vi "运维调试_总磷总氮.vi"() -> ()   [LabVIEW 2016, in "斯坦道总磷总氮.lvlib"]
uses:
  <vilib>/Utility/miscctls.llb/LVPointTypeDef.ctl
  <vilib>/Utility/config.llb/NI_LVConfig.lvlib
  <vilib>/ptbypt/NI_PtbyPt.lvlib
panel:
  in  "定时设置":cluster{"启动":bool, "控制命令":T1, "测量参数":T2}(xcontrol)
  in  "总磷参数设置":bool
  in  "总氮参数设置":bool
  in  "模块启用":bool
  in  "串口设置":bool
  in  "备用系数一键写入":bool
  in  "公式一键写入":bool
  in  "流程路径":path=path "C:/Users/std/Documents/斯坦道流程文件/流程.xml"
  in  "曲线模型":cluster{"X^2":dbl, "X":dbl, "B":dbl, "r^2":dbl}(xcontrol)
  out "字符串 2":string
  in  "质控参数设置":bool
  in  "总氮自动测试量程配置":T3
  in  "总磷自动测试量程配置":T3
  out "温度2":sgl
  out "温度1":sgl
  out "ADC":sgl
  out "固件版本号":string
  in  "数组":string[](array[string])
  in  "备用系数写入":bool
  in  "备用系数读取":bool
  in  "备用系数":T4
  in  "量程切换阈值写入":bool
  in  "量程切换阈值读取":bool
  in  "量程切换阈值":cluster{"阈值":dbl, "标液浓度":dbl}
  in  "参数下拉列表":enum16{"总磷", "总氮"}(ring)
  in  "量程下拉列表":enum16{"低量程", "高量程"}(ring)
  in  "测量模式下拉列表":enum16{"水样测量", "零点核查", "跨度核查", "标样核查", "加标回收"}(ring)
  in  "公式":cluster{"X^2":dbl, "X":dbl, "b":dbl}
  in  "写公式":bool
  in  "读公式":bool
  in  "返回":bool
  in  "设置":bool
  out "序列号":string="序列号"
  out "总氮测量数据":T5(xcontrol)
  out "总磷测量数据":T5(xcontrol)
  out "集成报警信息":string
  out "总磷总氮运行状态":T6(xcontrol)
  in  "停止":bool
  in  "手动启动":bool
  in  "单步测试":bool
  in  "总磷氨氮调试":u16[](xcontrol)
  out "F3":sgl format="%#.6f"
  out "F2":sgl format="%#.6f"
  out "F1":sgl format="%#.6f"
  out "F0":sgl format="%#.6f"
  out "多列列表框":i32(listbox)
  # "参数设置"
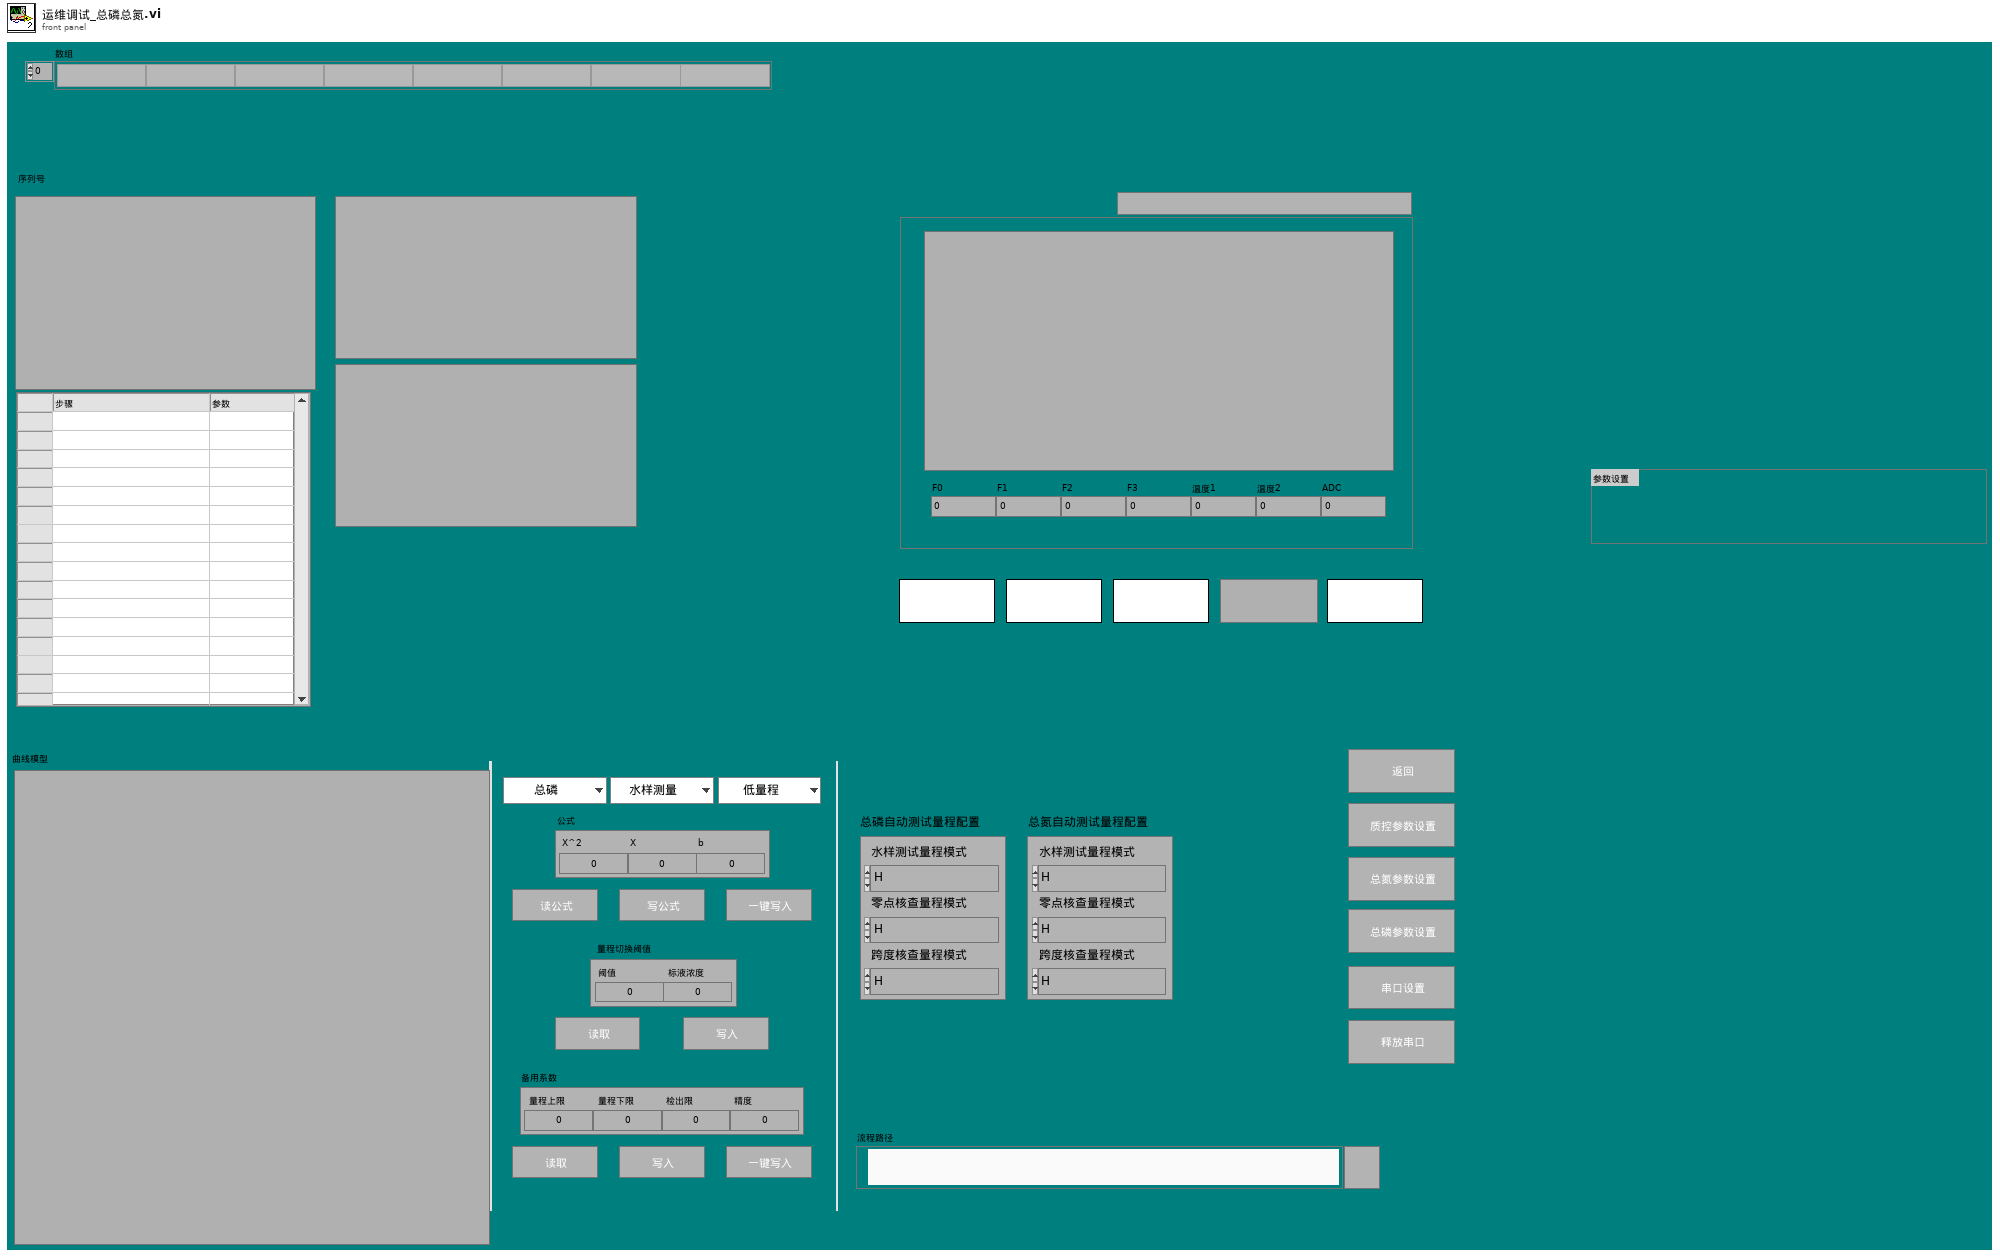
[diagram p1: front panel]
types:
  T1 = typedef "定时设置.xctl/国标控制命令.ctl" = enum16{"启动测量", "标样核查", "零点核查", "跨度核查", "空白测试", "平行样测试", "加标回收", "空白校准", "标样校准", "初始化（清洗）", "停止测试", "仪器重启", "校时", "模式设置", "测量间隔设置"}
  T2 = typedef "定时设置.xctl/测量参数.ctl" = u16
  T3 = cluster{"水样测试量程模式":enum16{"H", "L", "AUTO"}, "空白核查量程模式":enum16{"H", "L", "AUTO"}, "跨度核查量程模式":enum16{"H", "L", "AUTO"}}
  T4 = cluster{"量程上限":dbl, "量程下限":dbl, "检出限":dbl, "精度":dbl}
  T5 = cluster{"flowid":u16, "测量精度":u16, "测量数据区":cluster{"因子编码":u32, "单位":u16, "标样参考值":sgl, "水样数据时间":timestamp, "水样实测值":sgl, "水样数据标识":string, "标样数据时间":timestamp, "标样实测值":sgl, "标样数据标识":string, "空白数据时间":timestamp, "空白实测值":sgl, "空白数据标识":string, "零点核查数据时间":timestamp, "零点核查实测值":sgl, "零点核查数据标识":string, "跨度核查数据时间":timestamp, "跨度核查实测值":sgl, "跨度核查数据标识":string, "加标回收数据时间":timestamp, "加标回收实测值":sgl, "加标回收数据标识":string, "平行样数据时间":timestamp, "平行样实测值":sgl, "平行样数据标识":string, "F0":sgl, "F1":sgl, "F2":sgl, "F3":sgl, "F4":sgl, "F5":sgl, "F6":sgl, "F7":sgl, "温度":sgl, "湿度":sgl, "X值":sgl}}
  T6 = cluster{"系统时间":timestamp, "工作状态":enum16{"空闲", "水样测试", "标样核查", "零点核查", "跨度核查", "空白测试", "平行样测试", "加标回收", "空白校准", "标样校准", "初始化（清洗）"}, "测量模式":enum16{"待机", "连续模式", "周期模式", "定点模式", "受控模式", "手动模式"}, "告警代码":u16, "故障代码":u16, "日志代码":u16, "软件版本":u16, "F0":sgl, "F1":sgl, "F2":sgl, "F3":sgl, "T":sgl, "H":sgl, "id":u16, "flowid":u16, "量程":u16, "总磷控温温度1":sgl, "营养盐控温温度2":sgl, "ADC":sgl}
  T7 = cluster{"时间源选择":enum16{"系统时间源", "仪器时间源"}, "外部时间源":timestamp}
  T8 = enum16{"空闲", "水样测试", "标样核查", "零点核查", "跨度核查", "空白测试", "平行样测试", "加标回收", "空白校准", "标样校准", "初始化（清洗）"}
  T9 = enum32{"Bad", "Idle", "Run top level", "Running"}
  T10 = typedef "定时设置.xctl/周期模式设置.ctl" = enum16{"不启用", "定点模式", "间隔模式"}
  T11 = typedef "定时设置.xctl/定点周期设置.ctl" = cluster{"启动命令":T12, "启动命令 2":T12, "启动命令 3":T12, "启动命令 4":T12, "启动命令 5":T12, "启动命令 6":T12, "启动命令 7":T12, "启动命令 8":T12, "启动命令 9":T12, "启动命令 10":T12, "启动命令 11":T12, "启动命令 12":T12, "启动命令 13":T12, "启动命令 14":T12, "启动命令 15":T12, "启动命令 16":T12, "启动命令 17":T12, "启动命令 18":T12, "启动命令 19":T12, "启动命令 20":T12, "启动命令 21":T12, "启动命令 22":T12, "启动命令 23":T12, "启动命令 24":T12}
  T12 = typedef "定时设置.xctl/启动命令选择.ctl" = u16
  T13 = typedef "定时设置.xctl/间隔启动设置.ctl" = cluster{"启动命令":T12, "启动间隔":dbl, "启动次数":i32}
  T14 = cluster{"周期模式":T10, "定点周期":T11, "间隔启动":T13, "测量参数":T2}
  T15 = typedef "NI_LVConfig.lvlib/Config Data RefNum.ctl" = refnum<k1>
  T16 = typedef "LVPointTypeDef.ctl" = cluster{"Horizontal":i16, "Vertical":i16}
  T17 = cluster{"因子编码":u32, "单位":u16, "标样参考值":sgl, "水样数据时间":timestamp, "水样实测值":sgl, "水样数据标识":string, "标样数据时间":timestamp, "标样实测值":sgl, "标样数据标识":string, "空白数据时间":timestamp, "空白实测值":sgl, "空白数据标识":string, "零点核查数据时间":timestamp, "零点核查实测值":sgl, "零点核查数据标识":string, "跨度核查数据时间":timestamp, "跨度核查实测值":sgl, "跨度核查数据标识":string, "加标回收数据时间":timestamp, "加标回收实测值":sgl, "加标回收数据标识":string, "平行样数据时间":timestamp, "平行样实测值":sgl, "平行样数据标识":string, "F0":sgl, "F1":sgl, "F2":sgl, "F3":sgl, "F4":sgl, "F5":sgl, "F6":sgl, "F7":sgl, "温度":sgl, "湿度":sgl, "X值":sgl}
  T18 = cluster{"参数下拉列表":enum16{"总磷", "总氮"}, "测量模式下拉列表":enum16{"水样测量", "零点核查", "跨度核查", "标样核查", "加标回收"}, "量程下拉列表":enum16{"低量程", "高量程"}}
  T19 = cluster{"启动模式":enum16{"跨度核查", "水样测量", "空白核查", "标样核查", "加标回收"}, "启动参数":u16, "量程":enum16{"低量程", "高量程"}}
  T20 = cluster{"时间标识":timestamp, "设备":string, "日志信息":string, "流程参数":string}
  T21 = cluster{"时间标识":timestamp, "设备":string, "日志信息":string}
  T22 = typedef "LVRowAndColumnUnsignedTypeDef.ctl" = cluster{"Row":u32, "Column":u32}
  T23 = cluster{"站号":u16, "量程切换":enum32{"H", "L", "AUTO"}, "控制命令":enum16{"启动测量", "标样核查", "零点核查", "跨度核查", "空白测试", "平行样测试", "加标回收", "空白校准", "标样校准", "初始化（清洗）", "停止测试", "仪器重启", "校时", "模式设置", "测量间隔设置"}, "模式设置":enum16{"待机", "连续模式", "周期模式", "定点模式", "受控模式", "手动模式"}, "测量间隔":u16}
  T24 = cluster{"总磷跨度值":dbl, "总磷零点标准液浓度":dbl, "总磷跨度标准液浓度":dbl, "总磷标准液标准浓度":dbl, "总氮跨度值":dbl, "总氮零点标准液浓度":dbl, "总氮跨度标准液浓度":dbl, "总氮标准液标准浓度":dbl}
  T25 = cluster{"确定":bool, "总磷跨度值":dbl, "总磷零点标准液浓度":dbl, "总磷跨度标准液浓度":dbl, "总磷标准液标准浓度":dbl, "总氮跨度值":dbl, "总氮零点标准液浓度":dbl, "总氮跨度标准液浓度":dbl, "总氮标准液标准浓度":dbl}
  T26 = cluster{"测量量程":dbl, "测量精度":dbl, "测量间隔":dbl, "消解温度":dbl, "消解时长":dbl, "空白校准时间":timestamp, "曲线截距":dbl, "曲线斜率":dbl, "测量检出限":dbl, "测量信号值":dbl, "线性相关系数":dbl, "二次多项式系数":dbl, "标样校准时间":timestamp, "稀释倍数":dbl, "三项式系数":dbl, "空白标定系数":dbl, "量程系数":dbl, "F0/ORPA":dbl, "F1/ORPB":dbl, "F2/ORPK":dbl, "F3":dbl, "F4":dbl, "F5":dbl, "F6":dbl, "F7":dbl, "X0/滴定数":dbl, "量程":dbl}
  T27 = cluster{"确定":bool, "测量量程":dbl, "测量精度":dbl, "测量间隔":dbl, "消解温度":dbl, "消解时长":dbl, "空白校准时间":timestamp, "曲线截距":dbl, "曲线斜率":dbl, "测量检出限":dbl, "测量信号值":dbl, "线性相关系数":dbl, "二次多项式系数":dbl, "标样校准时间":timestamp, "稀释倍数":dbl, "三项式系数":dbl, "空白标定系数":dbl, "量程系数":dbl, "F0/ORPA":dbl, "F1/ORPB":dbl, "F2/ORPK":dbl, "F3":dbl, "F4":dbl, "F5":dbl, "F6":dbl, "F7":dbl, "X0/滴定数":dbl, "量程":dbl}
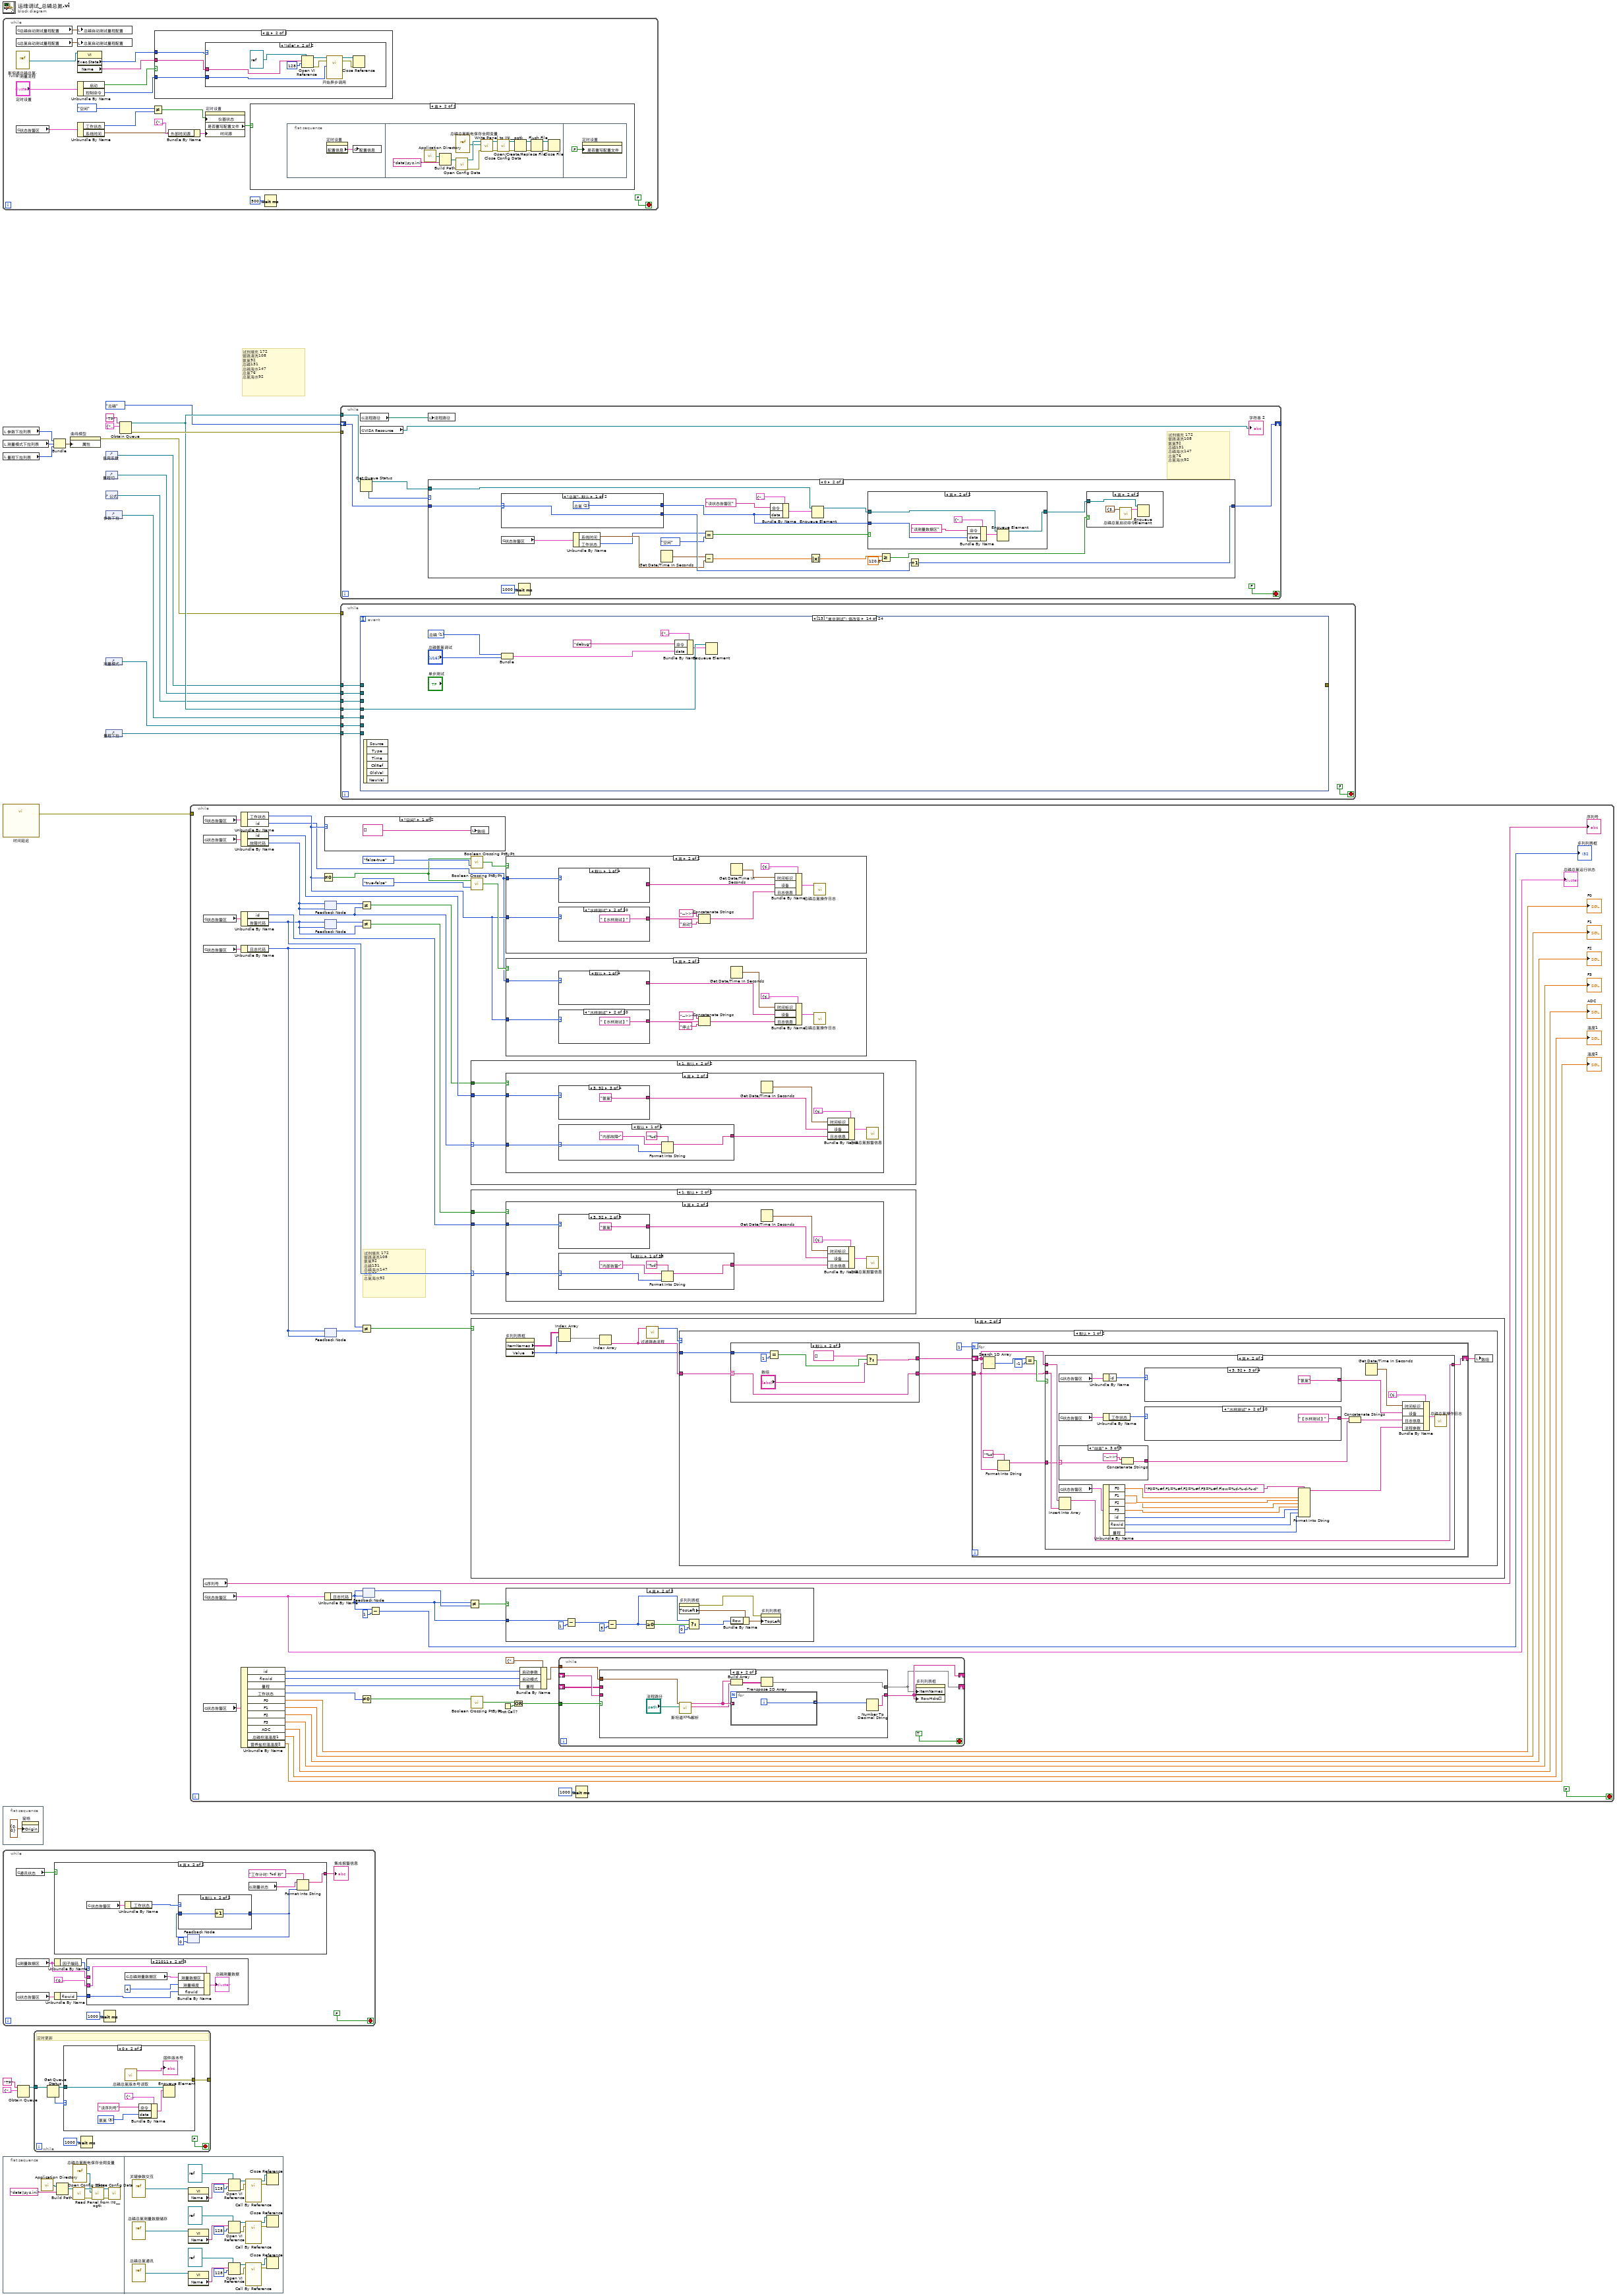
[diagram p0: block diagram]
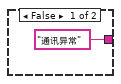
[diagram p3: hidden frame]
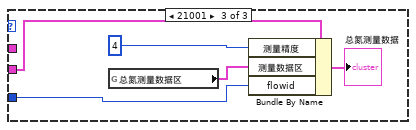
[diagram p6: hidden frame]
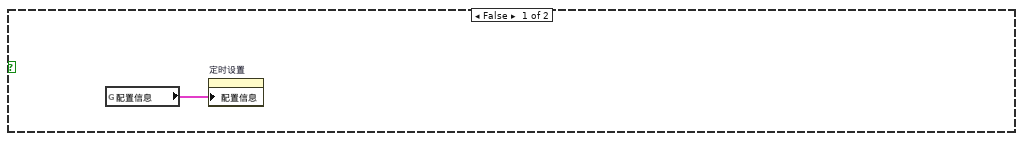
[diagram p7: hidden frame]
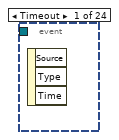
[diagram p10: hidden frame]
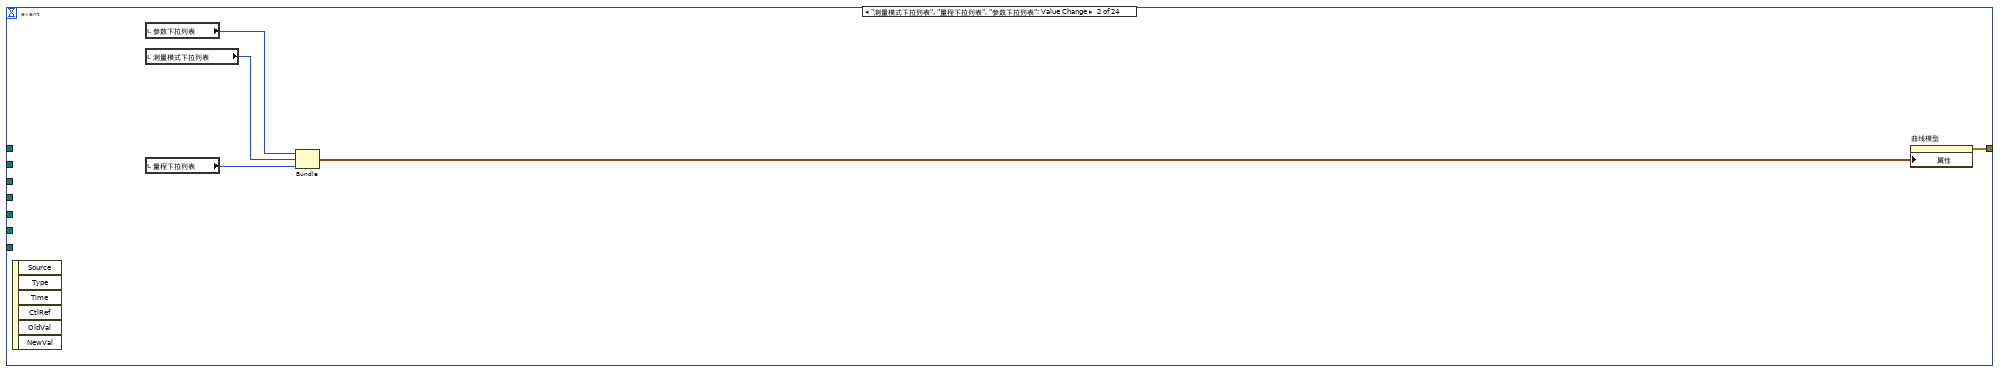
[diagram p11: hidden frame]
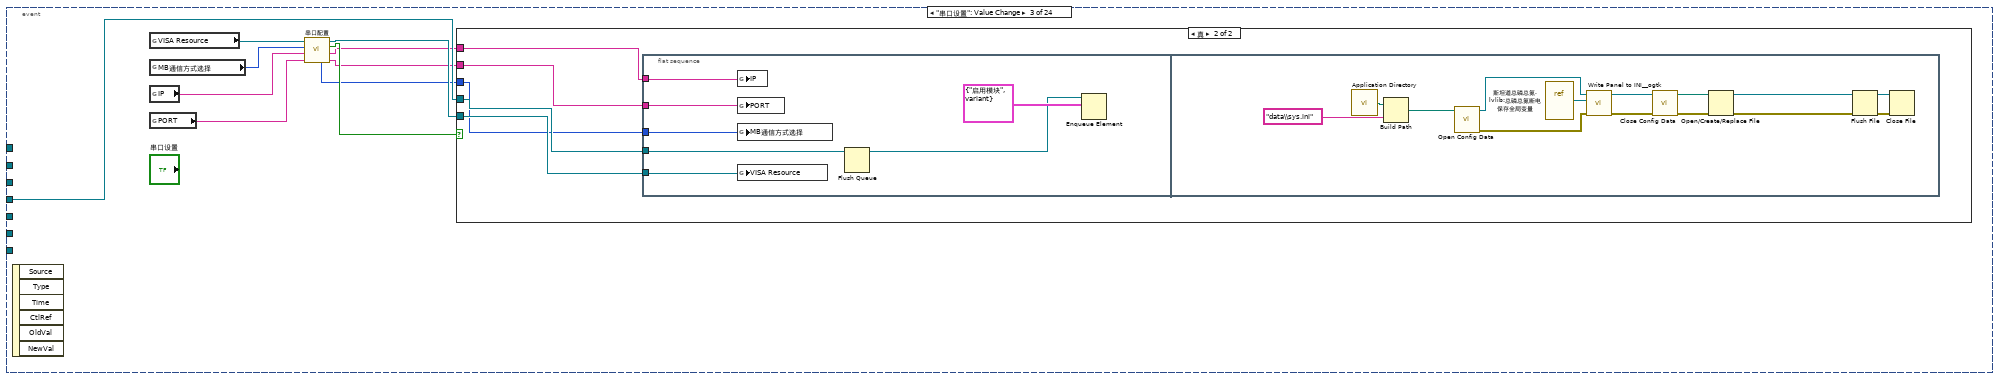
[diagram p12: hidden frame]
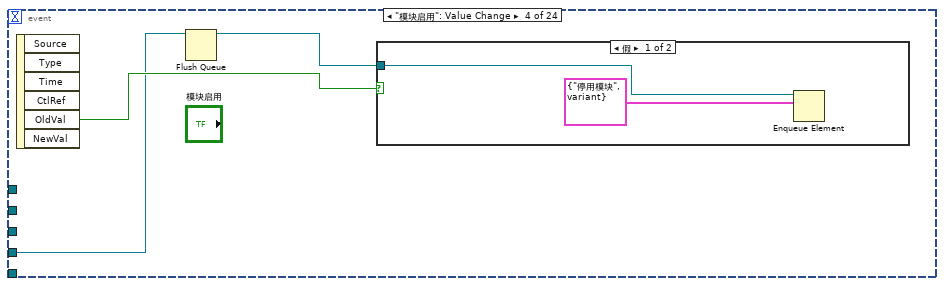
[diagram p14: hidden frame]
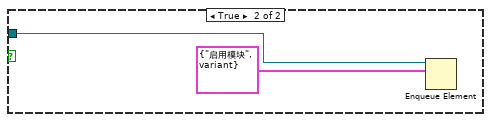
[diagram p15: hidden frame]
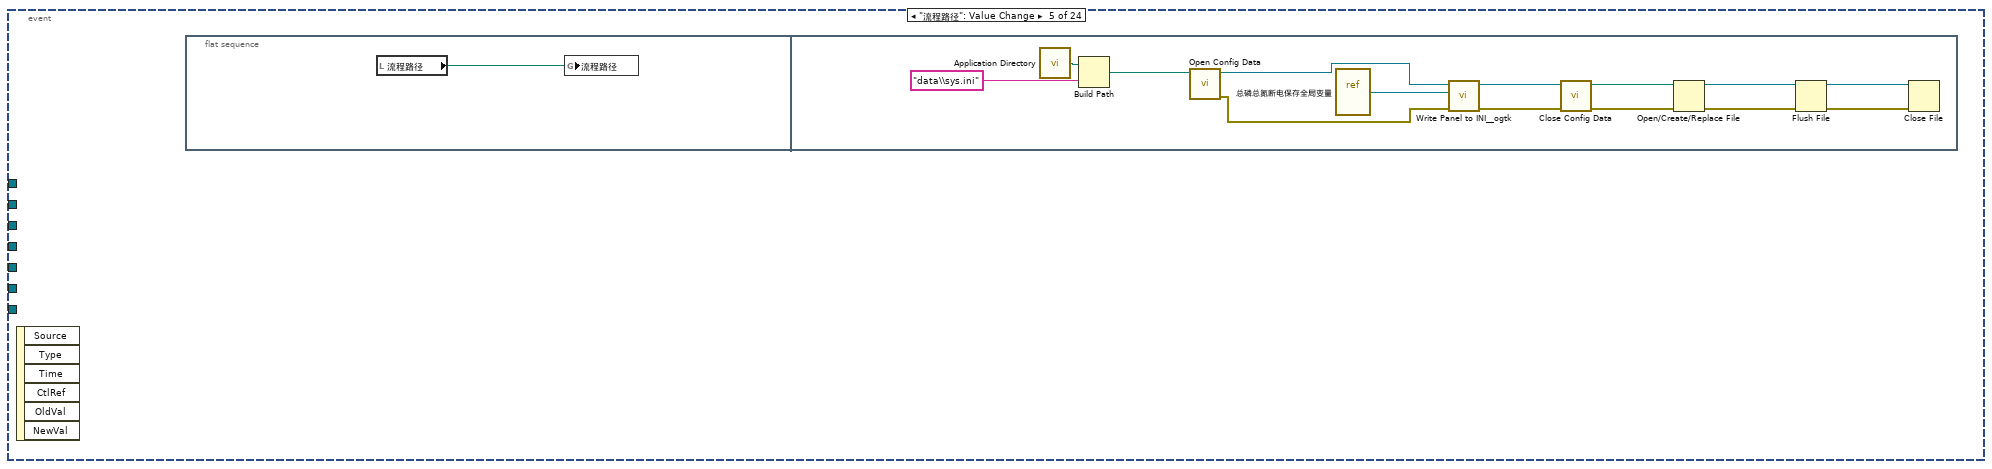
[diagram p16: hidden frame]
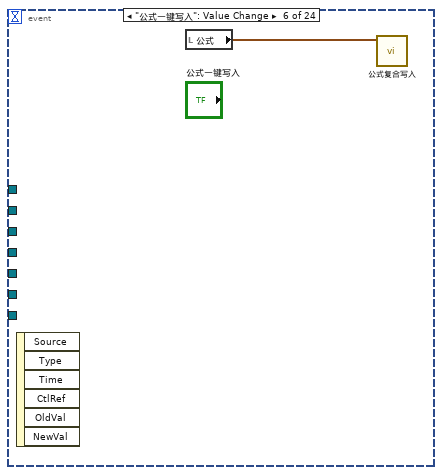
[diagram p17: hidden frame]
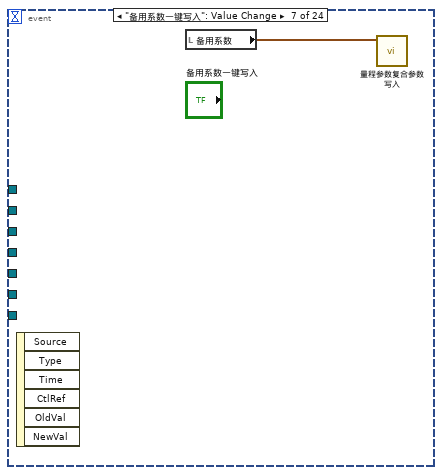
[diagram p18: hidden frame]
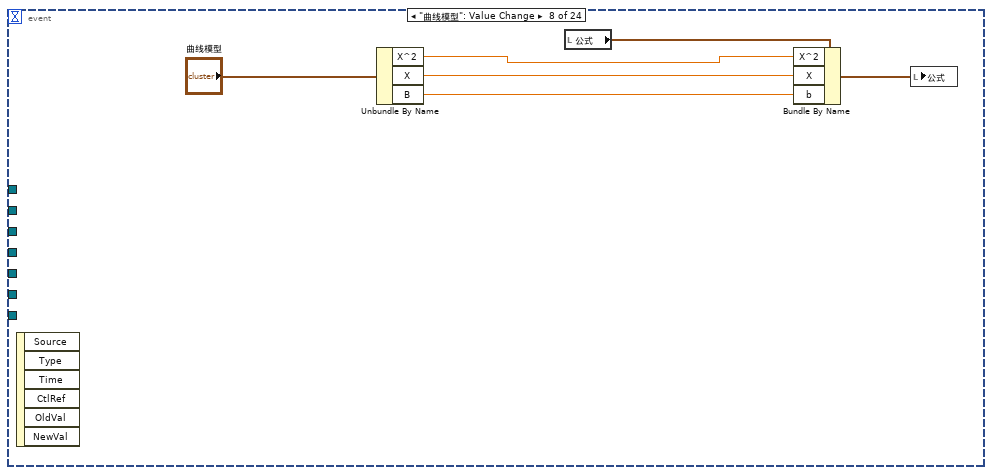
[diagram p19: hidden frame]
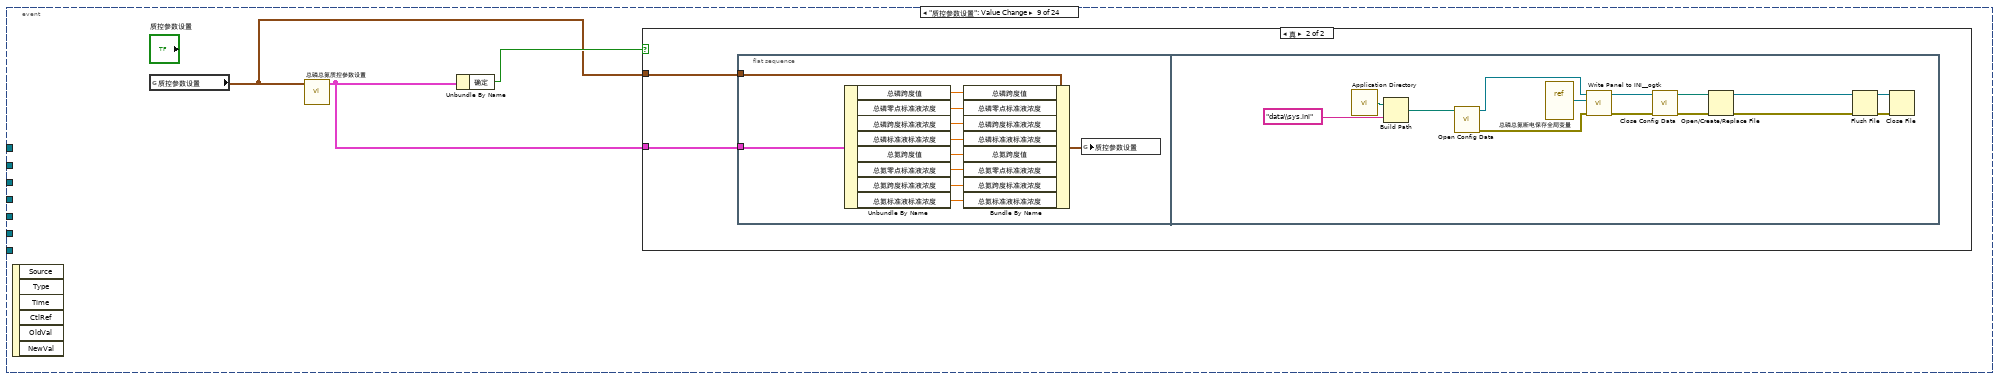
[diagram p20: hidden frame]
diagram:
  # "试剂填充 172 \n管路清洗108\n氨氮92\n总磷131\n总磷海水147\n总氮76\n总氮海水92"
  n1 = while {
    stop <- FALSE stop-if-true
    n2 = global read "总磷总氮断电保存全局变量.vi" "总磷自动测试量程配置"() -> (w35:T3)
    n3 = global read "总磷总氮断电保存全局变量.vi" "总氮自动测试量程配置"() -> (w36:T3)
    n4 = vi-ref "斯坦道总磷总氮.lvlib:测量流程.vi"() -> (w34:refnum<vi>)
    n5 = global read "VAR总磷总氮全局变量.vi" "状态告警区"() -> (w28:T6)
    n6 = local write "总磷自动测试量程配置"(w35) -> ()
    n7 = local write "总氮自动测试量程配置"(w36) -> ()
    n8 = property class="VI"(reference=w34) -> ("Exec.State"=w32:T9, "Name"=w33:string)  [unwired: 1 in, 2 out]
    n9 = Unbundle By Name("定时设置") -> ("启动"=w30:bool, "控制命令"=w29:T1)
    n10 = Unbundle By Name(w28) -> ("工作状态"=w27:T8, "系统时间"=w22:timestamp)
    n11 = Not Equal?(x=T8."空闲", y=w27) -> (x != y?=w25:bool)
    n12 = case shown="真" w30 {
      tunnel: w33 -> [_ w58]
      tunnel: w29 -> [_ w57]
      tunnel: w32 -> [_ w56]
      frame False {
      }
      frame True {
        n13 = case shown="\"Idle\"" w56 {
          tunnel: w58 -> [_ w62]
          tunnel: w57 -> [_ w59]
          frame "Bad", Default {
          }
          frame "Idle" {
            n14 = Open VI Reference(type specifier VI Refnum (for type only)=refnum<vi> refnum, vi path=w62, options=128 ("选项")) -> (vi reference=w63:refnum<vi>, error out=w64:errorcluster)  [unwired: 3 in]
            n15 = call-by-ref "开始异步调用"(reference=w63, error in=w64, "控制命令"=w59) -> (reference out=w65:refnum<vi>, error out=w66:errorcluster)  [unwired: 11 in]
            n16 = Close Reference(reference=w65, error in (no error)=w66) -> ()  [unwired: 1 out]
          }
        }
      }
    }
    n17 = Bundle By Name(cluster=T7 {"时间源选择"=enum."仪器时间源", "外部时间源"=timestamp(0 s since 1904-01-01)} ("时间源"), "外部时间源"=w22) -> (w21:T7)
    n18 = property on="定时设置" class="定时设置 (严格)"("仪器状态"=w25, "时间源"=w21) -> ("是否重写配置文件"=w24:bool)  [unwired: 2 in, 2 out]
    n19 = case shown="真" w24 {
      frame False {
        n20 = global read "总磷总氮断电保存全局变量.vi" "配置信息"() -> (w39:T14)
        n21 = property on="定时设置" class="定时设置 (严格)"("配置信息"=w39) -> ()  [unwired: 2 in, 2 out]
      }
      frame True {
        n22 = flat-sequence {
          frame #0 {
            n23 = property on="定时设置" class="定时设置 (严格)"() -> ("配置信息"=w40:T14)  [unwired: 2 in, 2 out]
            n24 = global write "总磷总氮断电保存全局变量.vi" "配置信息"(w40) -> ()
          }
          frame #1 {
            n25 = call <vilib>:"Application Directory.vi"() -> ("Application Directory"=w54:path)
            n26 = Build Path(base path=w54, name or relative path="data\\sys.ini" ("名称或相对路径")) -> (appended path=w52:path)
            n27 = vi-ref "总磷总氮断电保存全局变量.vi"() -> (w50:refnum<vi>)
            n28 = call <vilib>:"Open Config Data.vi"("configuration file path"=w52) -> ("error out"=w48:errorcluster, "refnum"=w51:T15)  [unwired: 8 in, 1 out]
            n29 = call <userlib>:"Write Panel to INI__ogtk.vi"("error in (no error)"=w48, "VI ref"=w50, "refnum"=w51) -> ("error out"=w47:errorcluster, "refnum out"=w49:T15)  [unwired: 7 in]
            n30 = call <vilib>:"Close Config Data.vi"("error in (no error)"=w47, "refnum"=w49) -> ("error out"=w42:errorcluster, "file path"=w41:path)  [unwired: 8 in]
            n31 = Open/Create/Replace File(file path (use dialog)=w41, error in=w42) -> (refnum out=w45:refnum<file>, error out=w46:errorcluster)  [unwired: 4 in, 1 out]
            n32 = Flush File(refnum=w45, error in=w46) -> (refnum out=w44:refnum<file>, error out=w43:errorcluster)
            n33 = Close File(refnum=w44, error in=w43) -> ()  [unwired: 2 out]
          }
          frame #2 {
            n34 = property on="定时设置" class="定时设置 (严格)"("是否重写配置文件"=FALSE) -> ()  [unwired: 2 in, 2 out]
          }
        }
      }
    }
    n35 = Wait (ms)(milliseconds to wait=u32 500 ("等待时间（毫秒）")) -> ()  [unwired: 1 out]
  }
  n36 = local read "参数下拉列表"() -> (w2:enum16{"总磷", "总氮"})
  n37 = local read "测量模式下拉列表"() -> (w3:enum16{"水样测量", "零点核查", "跨度核查", "标样核查", "加标回收"})
  n38 = local read "量程下拉列表"() -> (w1:enum16{"低量程", "高量程"})
  n39 = call "时间延迟"() -> ("error out"=w9:errorcluster)  [unwired: 11 in]
  n40 = flat-sequence {
    frame #0 {
      n41 = property on="窗格" class="Pane"("Origin"=T16 {"Horizontal"=0, "Vertical"=0} ("原点")) -> ()  [unwired: 2 in, 2 out]
    }
  }
  n42 = while {
    stop <- FALSE stop-if-true
    n43 = global read "VAR总磷总氮全局变量.vi" "通讯状态"() -> (w72:bool)
    n44 = global read "VAR总磷总氮全局变量.vi" "测量数据区"() -> (w74:T17)
    n45 = global read "VAR总磷总氮全局变量.vi" "状态告警区"() -> (w70:T6)
    n46 = case shown="真" w72 {
      tunnel: ["通讯异常" ("集成报警信息") w79] -> w71
      frame False {
      }
      frame True {
        n47 = global read "VAR总磷总氮全局变量.vi" "状态告警区"() -> (w85:T6)
        n48 = Unbundle By Name(w85) -> ("工作状态"=w84:T8)
        n49 = feedback #1(0) -> (w82:i32)
        n50 = case shown="默认" w84 {
          tunnel: w82 -> [_ w87]
          tunnel: [_ w86] -> w80
          frame "空闲" {
          }
          frame Default {
            n51 = Increment(x=w87) -> (x+1=w86:i32)
          }
        }
        n52 = feedback-in #1(w80) -> ()
        n53 = global read "VAR总磷总氮全局变量.vi" "测量状态"() -> (w78:string)
        n54 = Format Into String(format string="工作计时: %d 秒" ("格式字符串"), initial string=w78, w80) -> (resulting string=w79:string)  [unwired: 1 in, 1 out]
      }
    }
    "集成报警信息" <- w71
    n55 = Unbundle By Name(w74) -> ("因子编码"=w73:u32)
    n56 = Unbundle By Name(w70) -> ("flowid"=w69:u16)
    n57 = case shown="21011" w73 {
      tunnel: w74 -> [_ _ _]
      tunnel: w69 -> [_ w90 w96]
      tunnel: T5 {"flowid"=0, "测量精度"=0, "测量数据区"={"因子编码"=0, "单位"=0, "标样参考值"=0.0, "水样数据时间"=timestamp(0 s since 1904-01-01), "水样实测值"=0.0, "水样数据标识"="", "标样数据时间"=timestamp(0 s since 1904-01-01), "标样实测值"=0.0, "标样数据标识"="", "空白数据时间"=timestamp(0 s since 1904-01-01), "空白实测值"=0.0, "空白数据标识"="", "零点核查数据时间"=timestamp(0 s since 1904-01-01), "零点核查实测值"=0.0, "零点核查数据标识"="", "跨度核查数据时间"=timestamp(0 s since 1904-01-01), "跨度核查实测值"=0.0, "跨度核查数据标识"="", "加标回收数据时间"=timestamp(0 s since 1904-01-01), "加标回收实测值"=0.0, "加标回收数据标识"="", "平行样数据时间"=timestamp(0 s since 1904-01-01), "平行样实测值"=0.0, "平行样数据标识"="", "F0"=0.0, "F1"=0.0, "F2"=0.0, "F3"=0.0, "F4"=0.0, "F5"=0.0, "F6"=0.0, "F7"=0.0, "温度"=0.0, "湿度"=0.0, "X值"=0.0}} ("总氮测量数据") -> [_ w89 w95]
      frame Default {
      }
      frame 21011 {
        n58 = global read "VAR总磷总氮全局变量.vi" "总磷测量数据区"() -> (w88:T17)
        n59 = Bundle By Name(cluster=w89, "测量数据区"=w88, "测量精度"=u16 4, "flowid"=w90) -> (→"总磷测量数据":T5)
      }
      frame 21001 {
        n60 = global read "VAR总磷总氮全局变量.vi" "总氮测量数据区"() -> (w93:T17)
        n61 = Bundle By Name(cluster=w95, "测量精度"=u16 4, "测量数据区"=w93, "flowid"=w96) -> (→"总氮测量数据":T5)
      }
    }
    n62 = Wait (ms)(milliseconds to wait=u32 1000 ("等待时间（毫秒）")) -> ()  [unwired: 1 out]
  }
  n63 = flat-sequence {
    frame #0 {
      n64 = call <vilib>:"Application Directory.vi"() -> ("Application Directory"=w105:path)
      n65 = Build Path(base path=w105, name or relative path="data\\sys.ini" ("名称或相对路径")) -> (appended path=w103:path)
      n66 = vi-ref "总磷总氮断电保存全局变量.vi"() -> (w101:refnum<vi>)
      n67 = call <vilib>:"Open Config Data.vi"("configuration file path"=w103) -> ("error out"=w99:errorcluster, "refnum"=w102:T15)  [unwired: 8 in, 1 out]
      n68 = call <userlib>:"Read Panel from INI__ogtk.vi"("error in (no error)"=w99, "VI ref"=w101, "refnum"=w102) -> ("error out"=w98:errorcluster, "refnum out"=w100:T15)  [unwired: 7 in]
      n69 = call <vilib>:"Close Config Data.vi"("error in (no error)"=w98, "refnum"=w100) -> ()  [unwired: 8 in, 2 out]
    }
    frame #1 {
      n70 = vi-ref "关键参数交互.vi"() -> (w106:refnum<vi>)
      n71 = vi-ref "总磷总氮测量数据储存.vi"() -> (w121:refnum<vi>)
      n72 = vi-ref "总磷总氮通讯.vi"() -> (w129:refnum<vi>)
      n73 = property class="VI"(reference=w106) -> ("Name"=w113:string)  [unwired: 1 in, 2 out]
      n74 = property class="VI"(reference=w121) -> ("Name"=w114:string)  [unwired: 1 in, 2 out]
      n75 = property class="VI"(reference=w129) -> ("Name"=w128:string)  [unwired: 1 in, 2 out]
      n76 = Open VI Reference(type specifier VI Refnum (for type only)=refnum<vi> refnum, vi path=w113, options=128 ("选项")) -> (vi reference=w111:refnum<vi>, error out=w109:errorcluster)  [unwired: 3 in]
      n77 = Open VI Reference(type specifier VI Refnum (for type only)=refnum<vi> refnum, vi path=w114, options=128 ("选项")) -> (vi reference=w116:refnum<vi>, error out=w118:errorcluster)  [unwired: 3 in]
      n78 = Open VI Reference(type specifier VI Refnum (for type only)=refnum<vi> refnum, vi path=w128, options=128 ("选项")) -> (vi reference=w126:refnum<vi>, error out=w124:errorcluster)  [unwired: 3 in]
      n79 = call-by-ref "?"(reference=w111, error in=w109) -> (reference out=w107:refnum<vi>, error out=w108:errorcluster)  [unwired: 12 in]
      n80 = call-by-ref "?"(reference=w116, error in=w118) -> (reference out=w120:refnum<vi>, error out=w119:errorcluster)  [unwired: 12 in]
      n81 = call-by-ref "?"(reference=w126, error in=w124) -> (reference out=w122:refnum<vi>, error out=w123:errorcluster)  [unwired: 12 in]
      n82 = Close Reference(reference=w107, error in (no error)=w108) -> ()  [unwired: 1 out]
      n83 = Close Reference(reference=w120, error in (no error)=w119) -> ()  [unwired: 1 out]
      n84 = Close Reference(reference=w122, error in (no error)=w123) -> ()  [unwired: 1 out]
    }
  }
  n85 = Obtain Queue(name (unnamed)="TP" ("名称（未命名）"), element data type=cluster{"命令":string, "data":variant} {"命令"="", "data"=variant}) -> (queue out=w6:refnum<queue>)  [unwired: 3 in, 2 out]
  n86 = while {
    tunnel: w6 -> [w134]
    tunnel: [w132] -> _
    stop <- FALSE stop-if-true
    # "定时更新"
    n87 = Get Queue Status(queue=w134) -> (queue out=w131:refnum<queue>, # elements in queue=w130:i32)  [unwired: 2 in, 6 out]
    n88 = case shown="0" w130 {
      tunnel: w131 -> [_ w139]
      tunnel: [_ w136] -> w132
      frame Default {
      }
      frame 0 {
        w140 = u16 3 items=["总磷"=1, "氨氮"=3] ("站号")
        n89 = call "总磷总氮版本号读取.vi"() -> ("error out"=w136:errorcluster, "固件版本号"=→"固件版本号":string)  [unwired: 10 in]
        n90 = Bundle By Name(cluster=cluster{"命令":string, "data":variant} {"命令"="", "data"=variant} ("元素"), "命令"="读序列号", "data"=w140) -> (w138:cluster{"命令":string, "data":variant})
        n91 = Enqueue Element(queue=w139, element=w138) -> ()  [unwired: 2 in, 3 out]
      }
    }
    n92 = Wait (ms)(milliseconds to wait=u32 1000 ("等待时间（毫秒）")) -> ()  [unwired: 1 out]
  }
  n93 = Bundle("参数下拉列表"=w2, "测量模式下拉列表"=w3, "量程下拉列表"=w1) -> (w4:T18)  [unwired: 1 in]
  n94 = property on="曲线模型" class="曲线模型 (严格)"("属性"=w4) -> (error out=w5:errorcluster)  [unwired: 2 in, 1 out]
  n95 = control-ref of="备用系数"() -> (w10:refnum<vi>)
  n96 = control-ref of="量程切换阈值"() -> (w11:refnum<vi>)
  n97 = control-ref of="公式"() -> (w12:refnum<vi>)
  n98 = control-ref of="参数下拉列表"() -> (w14:refnum<vi>)
  n99 = control-ref of="测量模式下拉列表"() -> (w13:refnum<vi>)
  n100 = control-ref of="量程下拉列表"() -> (w15:refnum<vi>)
  n101 = Obtain Queue(name (unnamed)="TP" ("名称（未命名）"), element data type=cluster{"命令":string, "data":variant} {"命令"="", "data"=variant}) -> (queue out=w17:refnum<queue>, error out=w18:errorcluster)  [unwired: 3 in, 1 out]
  n102 = while {
    tunnel: w9 -> [_]
    stop <- FALSE stop-if-true
    # "试剂填充 172 \n管路清洗108\n氨氮92\n总磷131\n总磷海水147\n总氮76\n总氮海水92"
    n103 = global read "VAR总磷总氮全局变量.vi" "状态告警区"() -> (w163:T6)
    n104 = global read "VAR总磷总氮全局变量.vi" "状态告警区"() -> (w168:T6)
    n105 = global read "VAR总磷总氮全局变量.vi" "状态告警区"() -> (w173:T6)
    n106 = global read "VAR总磷总氮全局变量.vi" "状态告警区"() -> (w161:T6)
    n107 = global read "VAR总磷总氮全局变量.vi" "序列号"() -> (→"序列号":string)
    n108 = global read "VAR总磷总氮全局变量.vi" "状态告警区"() -> (w176:T6)
    "总磷总氮运行状态" <- w176
    n109 = global read "VAR总磷总氮全局变量.vi" "状态告警区"() -> (w184:T6)
    n110 = Unbundle By Name(w163) -> ("工作状态"=w144:T8, "id"=w143:u16)
    n111 = Unbundle By Name(w168) -> ("id"=w167:u16, "故障代码"=w164:u16)
    n112 = Unbundle By Name(w173) -> ("id"=w172:u16, "告警代码"=w169:u16)
    n113 = Unbundle By Name(w161) -> ("日志代码"=w160:u16)
    n114 = Unbundle By Name(w184) -> ("id"=w181:u16, "flowid"=w183:u16, "量程"=w182:u16, "工作状态"=w151:T8, "F0"=→"F0":sgl, "F1"=→"F1":sgl, "F2"=→"F2":sgl, "F3"=→"F3":sgl, "ADC"=→"ADC":sgl, "总磷控温温度1"=→"温度1":sgl, "营养盐控温温度2"=→"温度2":sgl)
    n115 = Not Equal To 0?(x=w144) -> (x != 0?=w146:bool)
    n116 = case shown="\"空闲\"" w144 {
      frame "空闲" {
        n117 = local write "数组"(string[] [] ("数组")) -> ()
      }
      frame "水样测试", Default {
      }
    }
    n118 = feedback #2(w164) -> (w165:u16)
    n119 = feedback-in #2(w164) -> ()
    n120 = feedback #3(w169) -> (w170:u16)
    n121 = feedback-in #3(w169) -> ()
    n122 = feedback #4(w160) -> (w162:u16)
    n123 = feedback-in #4(w160) -> ()
    n124 = Unbundle By Name(w176) -> ("日志代码"=w157:u16)
    n125 = Not Equal?(x=w165, y=w164) -> (x != y?=w166:bool)
    n126 = Not Equal?(x=w170, y=w169) -> (x != y?=w171:bool)
    n127 = Not Equal?(x=w160, y=w162) -> (x != y?=w159:bool)
    n128 = Not Equal To 0?(x=w151) -> (x != 0?=w186:bool)
    n129 = feedback-in #5(w157) -> ()
    n130 = feedback #5(w157) -> (w189:u16)
    n131 = Subtract(x=w157, y=1) -> (x-y=→"多列列表框":i32)
    n132 = Not Equal?(x=w157, y=w189) -> (x != y?=w188:bool)
    n133 = call <vilib>:"Boolean Crossing PtByPt.vi"("direction"=enum16{"either", "false-true", "true-false"}."false-true", "input"=w146) -> ("crossing"=w148:bool)  [unwired: 1 in]
    n134 = call <vilib>:"Boolean Crossing PtByPt.vi"("direction"=enum16{"either", "false-true", "true-false"}."true-false", "input"=w146) -> ("crossing"=w145:bool)  [unwired: 1 in]
    n135 = case shown="1, 默认" w164 {
      selector: w164 -> [_ w311]
      tunnel: w167 -> [_ w312]
      tunnel: w166 -> [_ w310]
      frame 0 {
      }
      frame 1, Default {
        n136 = case shown="真" w310 {
          tunnel: w312 -> [_ w319]
          tunnel: w311 -> [_ w314]
          frame False {
          }
          frame True {
            n137 = case shown="3, 92" w319 {
              tunnel: [_ "总磷" ("table输入") "氨氮" ("table输入") "总氮" ("table输入")] -> w315
              frame Default {
              }
              frame 1, 131 {
              }
              frame 3, 92 {
              }
              frame 2, 76 {
              }
            }
            n138 = case shown="默认" w314 {
              selector: w314 -> [w321 _ _ _ _ _]
              tunnel: [w320 "无故障" "电机故障" "温度故障" "通讯故障" "滴定故障"] -> w313
              frame Default {
                n139 = Format Into String(format string="%d" ("格式字符串"), initial string="内部故障-" ("工作状态"), w321) -> (resulting string=w320:string)  [unwired: 1 in, 1 out]
              }
              frame 0 {
              }
              frame 1 {
              }
              frame 2 {
              }
              frame 3 {
              }
              frame 4 {
              }
            }
            n140 = Get Date/Time In Seconds() -> (seconds since 1Jan1904=w316:timestamp)
            n141 = Bundle By Name(cluster=T21 {"时间标识"=timestamp(0 s since 1904-01-01), "设备"="", "日志信息"=""} ("data in"), "时间标识"=w316, "设备"=w315, "日志信息"=w313) -> (w317:T21)
            n142 = call "总磷总氮报警信息.vi"("data in"=w317) -> ()  [unwired: 10 in, 1 out]
          }
        }
      }
    }
    n143 = case shown="1, 默认" w169 {
      selector: w169 -> [_ w333]
      tunnel: w172 -> [_ w334]
      tunnel: w171 -> [_ w332]
      frame 0 {
      }
      frame 1, Default {
        n144 = case shown="真" w332 {
          tunnel: w334 -> [_ w341]
          tunnel: w333 -> [_ w335]
          frame False {
          }
          frame True {
            n145 = case shown="3, 92" w341 {
              tunnel: ["总磷" ("table输入") "氨氮" ("table输入") "总氮" ("table输入")] -> w337
              frame 1, 131 {
              }
              frame 3, 92 {
              }
              frame 2, 76, Default {
              }
            }
            n146 = case shown="默认" w335 {
              selector: w335 -> [w343 _ _ _ _ _ _ _ _ _ _ _ _ _ _ _ _ _ _ _ _ _ _ _ _ _ _ _ _ _ _ _ _ _ _ _ _ _]
              tunnel: [w342 "无告警" "缺试剂告警" "缺水样告警" "缺蒸馏水告警" "缺标液告警" "仪表漏液告警" "标定异常告警" "超量程告警" "加热异常" "低试剂预警" "超上限告警" "超下限告警" "仪表内部其他异常" "滴定异常告警" "电极异常告警" "量程切换告警" "参数设置告警" "PH电极电位异常" "电导率电极异常" "浊度光度异常" "溶解氧电极异常" "溶解氧光强异常" "温度异常告警" "PH异常告警" "溶解氧异常告警" "电导率异常告警" "浊度异常告警" "叶绿素异常告警" "藻密度异常告警" "蓝绿藻异常告警" "ORP异常告警" "氨氮异常告警" "清洁刷异常告警" "SD卡异常告警" "蓝牙异常告警" "WiFi异常告警" "流程异常告警"] -> w336
              frame Default {
                n147 = Format Into String(format string="%d" ("格式字符串"), initial string="内部告警-" ("工作状态"), w343) -> (resulting string=w342:string)  [unwired: 1 in, 1 out]
              }
              frame 0 {
              }
              frame 1 {
              }
              frame 2 {
              }
              frame 3 {
              }
              frame 4 {
              }
              frame 5 {
              }
              frame 6 {
              }
              frame 7 {
              }
              frame 8 {
              }
              frame 9 {
              }
              frame 10 {
              }
              frame 11 {
              }
              frame 12 {
              }
              frame 13 {
              }
              frame 14 {
              }
              frame 15 {
              }
              frame 16 {
              }
              frame 17 {
              }
              frame 18 {
              }
              frame 19 {
              }
              frame 20 {
              }
              frame 21 {
              }
              frame 22 {
              }
              frame 23 {
              }
              frame 24 {
              }
              frame 25 {
              }
              frame 26 {
              }
              frame 27 {
              }
              frame 28 {
              }
              frame 29 {
              }
              frame 30 {
              }
              frame 31 {
              }
              frame 32 {
              }
              frame 33 {
              }
              frame 34 {
              }
              frame 35 {
              }
              frame 36 {
              }
            }
            n148 = Get Date/Time In Seconds() -> (seconds since 1Jan1904=w338:timestamp)
            n149 = Bundle By Name(cluster=T21 {"时间标识"=timestamp(0 s since 1904-01-01), "设备"="", "日志信息"=""} ("data in"), "时间标识"=w338, "设备"=w337, "日志信息"=w336) -> (w339:T21)
            n150 = call "总磷总氮报警信息.vi"("data in"=w339) -> ()  [unwired: 10 in, 1 out]
          }
        }
      }
    }
    n151 = case shown="真" w159 {
      frame False {
      }
      frame True {
        n152 = property on="多列列表框" class="MCListbox (严格)"() -> ("ItemNames"=w241:string[][], "Value"=w237:i32)  [unwired: 2 in, 2 out]
        n153 = Index Array(array=w241, index (row)=w237) -> (element=w240:string[])  [unwired: 1 in]
        n154 = Index Array(array=w240) -> (element=w239:string)  [unwired: 1 in]
        n155 = call "过滤筛选流程.vi"("字符串"=w239) -> ("匹配后偏移量"=w238:i32)  [unwired: 10 in]
        n156 = case shown="默认" w238 {
          tunnel: w239 -> [w243 _]
          tunnel: w237 -> [w242 _]
          frame Default {
            n157 = case shown="默认" w243 {
              selector: w243 -> [w249 w256]
              tunnel: [w249 w256] -> w245
              tunnel: [string[] [] ("数组") w251] -> w244
              tunnel: w242 -> [_ w255]
              frame "读数" {
              }
              frame Default {
                n158 = Equal?(x=w255, y=1) -> (x = y?=w253:bool)
                n159 = Select(t=string[] [], s=w253, f="数组") -> (s? t:f=w251:string[])
              }
            }
            n160 = for {
              N: 1 -> [_]
              tunnel: w245 -> [w258]
              shift-right: [w257] -> w246
              shift-left: w244 -> [w259]
              n161 = Search 1D Array(1D array=w259, element=w258) -> (index of element=w262:i32)  [unwired: 1 in]
              n162 = Format Into String(format string="%s" ("格式字符串"), w258) -> (resulting string=w263:string)  [unwired: 2 in, 1 out]
              n163 = Equal?(x=w262, y=-1) -> (x = y?=w260:bool)
              n164 = case shown="真" w260 {
                tunnel: w263 -> [_ w271]
                tunnel: w259 -> [w265 w275]
                tunnel: w258 -> [_ w274]
                tunnel: [w265 w273] -> w257
                frame False {
                }
                frame True {
                  n165 = global read "VAR总磷总氮全局变量.vi" "状态告警区"() -> (w290:T6)
                  n166 = global read "VAR总磷总氮全局变量.vi" "状态告警区"() -> (w269:T6)
                  n167 = case shown="\"结束\"" w271 {
                    selector: w271 -> [w300 w303 w306]
                    tunnel: [w300 w302 w305] -> w270
                    frame Default {
                    }
                    frame "初始化" {
                      n168 = Concatenate Strings("-->>" ("字符串"), w303) -> (w302:string)
                    }
                    frame "结束" {
                      n169 = Concatenate Strings("-->>" ("字符串"), w306) -> (w305:string)
                    }
                  }
                  n170 = global read "VAR总磷总氮全局变量.vi" "状态告警区"() -> (w285:T6)
                  n171 = Insert Into Array(array=w275, new element=w274) -> (w273:string[])  [unwired: 1 in]
                  n172 = Unbundle By Name(w290) -> ("id"=w289:u16)
                  n173 = Unbundle By Name(w269) -> ("工作状态"=w268:T8)
                  n174 = Unbundle By Name(w285) -> ("F0"=w282:sgl, "F1"=w281:sgl, "F2"=w280:sgl, "F3"=w279:sgl, "id"=w278:u16, "flowid"=w277:u16, "量程"=w276:u16)
                  n175 = case shown="3, 92" w289 {
                    tunnel: [_ "总磷" ("table输入") "氨氮" ("table输入") "总氮" ("table输入")] -> w287
                    frame Default {
                    }
                    frame 1, 131 {
                    }
                    frame 3, 92 {
                    }
                    frame 2, 76 {
                    }
                  }
                  n176 = case shown="\"水样测试\"" w268 {
                    tunnel: [_ "【水样测试】" ("字符串") "【标样核查】" ("字符串") "【零点核查】" ("字符串") "【跨度核查】" ("字符串") "【空白测试】" ("字符串") "【平行样测试】" ("字符串") "【加标回收】" ("字符串") "【空白校准】" ("字符串") "【标样校准】" ("字符串")] -> w266
                    frame "空闲", Default {
                    }
                    frame "水样测试" {
                    }
                    frame "标样核查" {
                    }
                    frame "零点核查" {
                    }
                    frame "跨度核查" {
                    }
                    frame "空白测试" {
                    }
                    frame "平行样测试" {
                    }
                    frame "加标回收" {
                    }
                    frame "空白校准" {
                    }
                    frame "标样校准" {
                    }
                  }
                  n177 = Format Into String(format string="F0=%#f,F1=%#f,F2=%#f,F3=%#f,Flow=%d-%-d-%-d" ("格式字符串"), w282, w281, w280, w279, w278, w277, w276) -> (resulting string=w283:string)  [unwired: 2 in, 1 out]
                  n178 = Concatenate Strings(w266, w270) -> (w267:string)
                  n179 = Get Date/Time In Seconds() -> (seconds since 1Jan1904=w286:timestamp)
                  n180 = Bundle By Name(cluster=T20 {"时间标识"=timestamp(0 s since 1904-01-01), "设备"="", "日志信息"="", "流程参数"=""} ("data in"), "时间标识"=w286, "设备"=w287, "日志信息"=w267, "流程参数"=w283) -> (w288:T20)
                  n181 = call "总磷总氮操作日志.vi"("data in"=w288) -> ()  [unwired: 11 in]
                }
              }
            }
            n182 = local write "数组"(w246) -> ()
          }
          frame -1 {
          }
        }
      }
    }
    n183 = call <vilib>:"Boolean Crossing PtByPt.vi"("input"=w186) -> ("crossing"=w150:bool)  [unwired: 2 in]
    n184 = First Call?() -> (First Call?: T/F=w187:bool)
    n185 = case shown="真" w148 {
      tunnel: w144 -> [_ w216]
      tunnel: w143 -> [_ w215]
      frame False {
      }
      frame True {
        n186 = case shown="默认" w215 {
          tunnel: [_ "总磷" ("table输入") "氨氮" ("table输入") "总氮" ("table输入")] -> w219
          frame Default {
          }
          frame 1, 131 {
          }
          frame 3, 92 {
          }
          frame 2, 76 {
          }
        }
        n187 = case shown="\"水样测试\"" w216 {
          tunnel: [_ "【水样测试】" ("字符串") "【标样核查】" ("字符串") "【零点核查】" ("字符串") "【跨度核查】" ("字符串") "【空白测试】" ("字符串") "【平行样测试】" ("字符串") "【加标回收】" ("字符串") "【空白校准】" ("字符串") "【标样校准】" ("字符串")] -> w223
          frame "空闲", Default {
          }
          frame "水样测试" {
          }
          frame "标样核查" {
          }
          frame "零点核查" {
          }
          frame "跨度核查" {
          }
          frame "空白测试" {
          }
          frame "平行样测试" {
          }
          frame "加标回收" {
          }
          frame "空白校准" {
          }
          frame "标样校准" {
          }
        }
        n188 = Concatenate Strings("-->>" ("字符串"), w223, "启动" ("字符串")) -> (w222:string)
        n189 = Get Date/Time In Seconds() -> (seconds since 1Jan1904=w220:timestamp)
        n190 = Bundle By Name(cluster=T20 {"时间标识"=timestamp(0 s since 1904-01-01), "设备"="", "日志信息"="", "流程参数"=""} ("data in"), "时间标识"=w220, "设备"=w219, "日志信息"=w222) -> (w214:T20)
        n191 = call "总磷总氮操作日志.vi"("data in"=w214) -> ()  [unwired: 11 in]
      }
    }
    n192 = case shown="真" w145 {
      tunnel: w144 -> [_ w194]
      tunnel: w143 -> [_ w193]
      frame False {
      }
      frame True {
        n193 = case shown="默认" w193 {
          tunnel: [_ "总磷" ("table输入") "氨氮" ("table输入") "总氮" ("table输入")] -> w197
          frame Default {
          }
          frame 1, 131 {
          }
          frame 3, 92 {
          }
          frame 2, 76 {
          }
        }
        n194 = case shown="\"水样测试\"" w194 {
          tunnel: [_ "【水样测试】" ("字符串") "【标样核查】" ("字符串") "【零点核查】" ("字符串") "【跨度核查】" ("字符串") "【空白测试】" ("字符串") "【平行样测试】" ("字符串") "【加标回收】" ("字符串") "【空白校准】" ("字符串") "【标样校准】" ("字符串")] -> w201
          frame "空闲", Default {
          }
          frame "水样测试" {
          }
          frame "标样核查" {
          }
          frame "零点核查" {
          }
          frame "跨度核查" {
          }
          frame "空白测试" {
          }
          frame "平行样测试" {
          }
          frame "加标回收" {
          }
          frame "空白校准" {
          }
          frame "标样校准" {
          }
        }
        n195 = Concatenate Strings("-->>" ("字符串"), w201, "停止" ("字符串")) -> (w200:string)
        n196 = Get Date/Time In Seconds() -> (seconds since 1Jan1904=w198:timestamp)
        n197 = Bundle By Name(cluster=T20 {"时间标识"=timestamp(0 s since 1904-01-01), "设备"="", "日志信息"="", "流程参数"=""} ("data in"), "时间标识"=w198, "设备"=w197, "日志信息"=w200) -> (w192:T20)
        n198 = call "总磷总氮操作日志.vi"("data in"=w192) -> ()  [unwired: 11 in]
      }
    }
    n199 = case shown="真" w188 {
      tunnel: w157 -> [_ w406]
      frame False {
      }
      frame True {
        n200 = Subtract(x=w406, y=1) -> (x-y=w404:i32)
        n201 = Subtract(x=w404, y=5) -> (x-y=w408:i32)
        n202 = Greater Or Equal To 0?(x=w408) -> (x >= 0?=w407:bool)
        n203 = property on="多列列表框" class="MCListbox (严格)"() -> (error out=w412:errorcluster, "TopLeft"=w413:T22)  [unwired: 2 in, 1 out]
        n204 = Select(t=w408, s=w407, f=0) -> (s? t:f=w409:i32)
        n205 = Bundle By Name(cluster=w413, "Row"=w409) -> (w414:T22)
        n206 = property on="多列列表框" class="MCListbox (严格)"(error in=w412, "TopLeft"=w414) -> ()  [unwired: 1 in, 2 out]
      }
    }
    n207 = Or(x=w150, y=w187) -> (x .or. y?=w185:bool)
    n208 = Bundle By Name(cluster=T19 {"启动模式"=enum."跨度核查", "启动参数"=1, "量程"=enum."低量程"} ("参数簇"), "启动参数"=w181, "启动模式"=w183, "量程"=w182) -> (w175:T19)
    n209 = while {
      tunnel: w185 -> [w392]
      tunnel: w175 -> [w391]
      shift-right: [w386] -> _
      shift-left: _ -> [w388]
      shift-right: [w387] -> _
      shift-left: _ -> [w389]
      stop <- TRUE stop-if-true
      n210 = case shown="真" w392 {
        tunnel: [w394 w402] -> w387
        tunnel: [w393 w401] -> w386
        tunnel: w391 -> [_ w396]
        tunnel: w389 -> [w394 _]
        tunnel: w388 -> [w393 _]
        frame False {
        }
        frame True {
          n211 = call "斯坦道XML解析.vi"("添加的路径"="流程路径", "参数簇"=w396) -> ("步骤时间"=w397:string[], "步骤名"=w399:string[])  [unwired: 8 in]
          n212 = Build Array(w399, w397) -> (w398:string[][])
          n213 = for {
            tunnel: w399 -> [_] mode=indexing
            tunnel: [w403] -> w400 mode=indexing
            i -> [w403]
          }
          n214 = Transpose 2D Array(2D array=w398) -> (transposed array=w401:string[][])
          n215 = Number To Decimal String(number=w400) -> (decimal integer string=w402:string[])  [unwired: 1 in]
        }
      }
      n216 = property on="多列列表框" class="MCListbox (严格)"("ItemNames"=w386, "RowHdrs[]"=w387) -> ()  [unwired: 2 in, 2 out]
    }
    n217 = Wait (ms)(milliseconds to wait=u32 1000 ("等待时间（毫秒）")) -> ()  [unwired: 1 out]
  }
  n218 = while {
    tunnel: w17 -> [w421]
    tunnel: w18 -> [_]
    shift-right: [w419] -> _
    shift-left: enum16{"总磷", "总氮"}."总磷" ("枚举") -> [w420]
    stop <- FALSE stop-if-true
    # "试剂填充 172 \n管路清洗108\n氨氮92\n总磷131\n总磷海水147\n总氮76\n总氮海水92"
    n219 = global read "总磷总氮断电保存全局变量.vi" "流程路径"() -> (w418:path)
    n220 = global read "总磷总氮断电保存全局变量.vi" "VISA Resource"() -> (→"字符串 2":refnum<visa-resource-name>)
    n221 = Get Queue Status(queue=w421) -> (queue out=w416:refnum<queue>, # elements in queue=w415:i32)  [unwired: 2 in, 6 out]
    n222 = local write "流程路径"(w418) -> ()
    n223 = case shown="0" w415 {
      tunnel: w420 -> [w424 w444]
      tunnel: [w424 w443] -> w419
      tunnel: w416 -> [_ w442]
      frame Default {
      }
      frame 0 {
        n224 = case shown="\"总氮\", 默认" w444 {
          selector: w444 -> [w455 w457]
          tunnel: [w456 w458] -> w437
          tunnel: [w455 w457] -> w436
          frame "总氮", Default {
            w456 = u16 2 items=["总磷"=1, "总氮"=2] ("站号")
          }
          frame "总磷" {
            w458 = u16 1 items=["总磷"=1, "氨氮"=3] ("站号")
          }
        }
        n225 = global read "VAR总磷总氮全局变量.vi" "状态告警区"() -> (w428:T6)
        n226 = Unbundle By Name(w428) -> ("系统时间"=w435:timestamp, "工作状态"=w427:T8)
        n227 = Get Date/Time In Seconds() -> (seconds since 1Jan1904=w434:timestamp)
        n228 = Equal?(x=w427, y=T8."空闲") -> (x = y?=w425:bool)
        n229 = Subtract(x=w434, y=w435) -> (x-y=w433:dbl)
        n230 = Bundle By Name(cluster=cluster{"命令":string, "data":variant} {"命令"="", "data"=variant} ("元素"), "命令"="读状态告警区", "data"=w437) -> (w440:cluster{"命令":string, "data":variant})
        n231 = Absolute Value(x=w433) -> (abs(x)=w432:dbl)
        n232 = Enqueue Element(queue=w442, element=w440) -> (queue out=w438:refnum<queue>)  [unwired: 2 in, 2 out]
        n233 = case shown="真" w425 {
          tunnel: w438 -> [w445 w448]
          tunnel: w437 -> [_ w447]
          tunnel: [w445 w446] -> w429
          frame False {
          }
          frame True {
            n234 = Bundle By Name(cluster=cluster{"命令":string, "data":variant} {"命令"="", "data"=variant} ("元素"), "命令"="读测量数据区", "data"=w447) -> (w450:cluster{"命令":string, "data":variant})
            n235 = Enqueue Element(queue=w448, element=w450) -> (queue out=w446:refnum<queue>)  [unwired: 2 in, 2 out]
          }
        }
        n236 = Greater Or Equal?(x=w432, y=120.0) -> (x >= y?=w430:bool)
        n237 = Increment(x=w436) -> (x+1=w443:enum16{"总磷", "总氮"})
        n238 = case shown="真" w430 {
          tunnel: w429 -> [_ w453]
          frame False {
          }
          frame True {
            n239 = call "总磷总氮启动命令.vi"("参数"=T23 {"站号"=3, "量程切换"=enum."AUTO", "控制命令"=enum."校时", "模式设置"=enum."待机", "测量间隔"=0}) -> ("启动命令"=w452:cluster{"命令":string, "data":variant})  [unwired: 10 in]
            n240 = Enqueue Element(queue=w453, element=w452) -> ()  [unwired: 2 in, 3 out]
          }
        }
      }
    }
    n241 = Wait (ms)(milliseconds to wait=u32 1000 ("等待时间（毫秒）")) -> ()  [unwired: 1 out]
  }
  n242 = while {
    tunnel: w17 -> [w465]
    tunnel: w15 -> [w464]
    tunnel: w14 -> [w463]
    tunnel: w13 -> [w462]
    tunnel: w12 -> [w461]
    tunnel: w11 -> [w460]
    tunnel: w10 -> [w459]
    tunnel: w5 -> [_]
    stop <- FALSE stop-if-true
    n243 = event shown="[13] \"单步测试\": 值改变" {
      selector: _ -> [_ _ _ _ _ _ _ _ _ _ _ _ _ _ _ _ _ _ _ _ _ _ _ _]
      dyn-events: _ -> [_ _ _ _ _ _ _ _ _ _ _ _ _ _ _ _ _ _ _ _ _ _ _ _]
      timeout: _ -> [_ _ _ _ _ _ _ _ _ _ _ _ _ _ _ _ _ _ _ _ _ _ _ _]
      tunnel: w465 -> [_ _ w481 w509 _ _ _ _ _ _ _ _ w656 w665 w669 _ _ _ _ _ _ _ _ _]
      tunnel: w464 -> [_ _ _ _ _ _ _ _ _ _ _ _ _ _ _ _ _ _ w685 _ w728 w737 w745 w756]
      tunnel: w463 -> [_ _ _ _ _ _ _ _ _ _ _ _ _ _ _ _ _ _ w683 _ w726 w739 w751 w762]
      tunnel: w462 -> [_ _ _ _ _ _ _ _ _ _ _ _ _ _ _ _ _ _ w684 _ w727 w738 w744 w757]
      tunnel: w461 -> [_ _ _ _ _ _ _ _ _ _ _ _ _ _ _ _ _ _ w679 _ _ _ _ _]
      tunnel: w460 -> [_ _ _ _ _ _ _ _ _ _ _ _ _ _ _ _ _ _ _ _ w722 _ _ _]
      tunnel: w459 -> [_ _ _ _ _ _ _ _ _ _ _ _ _ _ _ _ _ _ _ _ _ _ w749 _]
      tunnel: [_ w467 _ _ _ _ _ _ _ _ _ _ _ _ _ _ _ _ _ _ _ _ _ _] -> _
      event Timeout {
        n244 = event-data() -> ()  [unwired: 1 in, 3 out]
      }
      event "测量模式下拉列表", "量程下拉列表", "参数下拉列表": Value Change {
        n245 = event-data() -> ()  [unwired: 1 in, 6 out]
        n246 = local read "参数下拉列表"() -> (w470:enum16{"总磷", "总氮"})
        n247 = local read "测量模式下拉列表"() -> (w469:enum16{"水样测量", "零点核查", "跨度核查", "标样核查", "加标回收"})
        n248 = local read "量程下拉列表"() -> (w471:enum16{"低量程", "高量程"})
        n249 = Bundle("参数下拉列表"=w470, "测量模式下拉列表"=w469, "量程下拉列表"=w471) -> (w468:T18)  [unwired: 1 in]
        n250 = property on="曲线模型" class="曲线模型 (严格)"("属性"=w468) -> (error out=w467:errorcluster)  [unwired: 2 in, 1 out]
      }
      event "串口设置": Value Change {
        n251 = event-data() -> ()  [unwired: 1 in, 6 out]
        n252 = global read "总磷总氮断电保存全局变量.vi" "VISA Resource"() -> (w478:refnum<visa-resource-name>)
        n253 = global read "总磷总氮断电保存全局变量.vi" "MB通信方式选择"() -> (w472:enum16{"串口", "TCP"})
        n254 = global read "总磷总氮断电保存全局变量.vi" "IP"() -> (w477:string)
        n255 = global read "总磷总氮断电保存全局变量.vi" "PORT"() -> (w476:string)
        n256 = call "串口配置.vi"("PORT"=w476, "IP"=w477, "MB通信方式选择"=w472, "请选择串口:"=w478) -> ("PORT 2"=w474:string, "IP 2"=w475:string, "确认 2"=w479:bool, "VISA资源名称 2"=w480:refnum<visa-resource-name>, "MB通信方式选择 2"=w473:enum16{"串口", "TCP"})  [unwired: 3 in]
        n257 = case shown="真" w479 {
          tunnel: w480 -> [_ w486]
          tunnel: w481 -> [_ w485]
          tunnel: w475 -> [_ w484]
          tunnel: w474 -> [_ w483]
          tunnel: w473 -> [_ w482]
          frame False {
          }
          frame True {
            n258 = flat-sequence {
              tunnel: w486 -> [w491]
              tunnel: w485 -> [w492]
              tunnel: w484 -> [w490]
              tunnel: w483 -> [w489]
              tunnel: w482 -> [w488]
              frame #0 {
                n259 = global write "总磷总氮断电保存全局变量.vi" "IP"(w490) -> ()
                n260 = global write "总磷总氮断电保存全局变量.vi" "PORT"(w489) -> ()
                n261 = global write "总磷总氮断电保存全局变量.vi" "MB通信方式选择"(w488) -> ()
                n262 = global write "总磷总氮断电保存全局变量.vi" "VISA Resource"(w491) -> ()
                n263 = Flush Queue(queue=w492) -> (queue out=w487:refnum<queue>)  [unwired: 1 in, 2 out]
                n264 = Enqueue Element(queue=w487, element=cluster{"命令":string, "data":variant} {"命令"="启用模块", "data"=variant} ("元素")) -> ()  [unwired: 2 in, 3 out]
              }
              frame #1 {
                n265 = call <vilib>:"Application Directory.vi"() -> ("Application Directory"=w507:path)
                n266 = Build Path(base path=w507, name or relative path="data\\sys.ini" ("名称或相对路径")) -> (appended path=w505:path)
                n267 = call <vilib>:"Open Config Data.vi"("configuration file path"=w505) -> ("error out"=w501:errorcluster, "refnum"=w504:T15)  [unwired: 8 in, 1 out]
                n268 = vi-ref "斯坦道总磷总氮.lvlib:总磷总氮断电保存全局变量.vi"() -> (w503:refnum<vi>)
                n269 = call <userlib>:"Write Panel to INI__ogtk.vi"("error in (no error)"=w501, "VI ref"=w503, "refnum"=w504) -> ("error out"=w500:errorcluster, "refnum out"=w502:T15)  [unwired: 7 in]
                n270 = call <vilib>:"Close Config Data.vi"("error in (no error)"=w500, "refnum"=w502) -> ("error out"=w495:errorcluster, "file path"=w494:path)  [unwired: 8 in]
                n271 = Open/Create/Replace File(file path (use dialog)=w494, error in=w495) -> (refnum out=w498:refnum<file>, error out=w499:errorcluster)  [unwired: 4 in, 1 out]
                n272 = Flush File(refnum=w498, error in=w499) -> (refnum out=w497:refnum<file>, error out=w496:errorcluster)
                n273 = Close File(refnum=w497, error in=w496) -> ()  [unwired: 2 out]
              }
            }
          }
        }
      }
      event "模块启用": Value Change {
        n274 = event-data() -> ("OldVal"=w510:bool)  [unwired: 1 in, 5 out]
        n275 = Flush Queue(queue=w509) -> (queue out=w508:refnum<queue>)  [unwired: 1 in, 2 out]
        n276 = case shown="假" w510 {
          tunnel: w508 -> [w511 w513]
          frame False {
            n277 = Enqueue Element(queue=w511, element=cluster{"命令":string, "data":variant} {"命令"="停用模块", "data"=variant} ("元素")) -> ()  [unwired: 2 in, 3 out]
          }
          frame True {
            n278 = Enqueue Element(queue=w513, element=cluster{"命令":string, "data":variant} {"命令"="启用模块", "data"=variant} ("元素")) -> ()  [unwired: 2 in, 3 out]
          }
        }
      }
      event "流程路径": Value Change {
        n279 = event-data() -> ()  [unwired: 1 in, 6 out]
        n280 = flat-sequence {
          frame #0 {
            n281 = local read "流程路径"() -> (w515:path)
            n282 = global write "总磷总氮断电保存全局变量.vi" "流程路径"(w515) -> ()
          }
          frame #1 {
            n283 = call <vilib>:"Application Directory.vi"() -> ("Application Directory"=w529:path)
            n284 = Build Path(base path=w529, name or relative path="data\\sys.ini" ("名称或相对路径")) -> (appended path=w527:path)
            n285 = call <vilib>:"Open Config Data.vi"("configuration file path"=w527) -> ("error out"=w523:errorcluster, "refnum"=w526:T15)  [unwired: 8 in, 1 out]
            n286 = vi-ref "总磷总氮断电保存全局变量.vi"() -> (w525:refnum<vi>)
            n287 = call <userlib>:"Write Panel to INI__ogtk.vi"("error in (no error)"=w523, "VI ref"=w525, "refnum"=w526) -> ("error out"=w522:errorcluster, "refnum out"=w524:T15)  [unwired: 7 in]
            n288 = call <vilib>:"Close Config Data.vi"("error in (no error)"=w522, "refnum"=w524) -> ("error out"=w517:errorcluster, "file path"=w516:path)  [unwired: 8 in]
            n289 = Open/Create/Replace File(file path (use dialog)=w516, error in=w517) -> (refnum out=w520:refnum<file>, error out=w521:errorcluster)  [unwired: 4 in, 1 out]
            n290 = Flush File(refnum=w520, error in=w521) -> (refnum out=w519:refnum<file>, error out=w518:errorcluster)
            n291 = Close File(refnum=w519, error in=w518) -> ()  [unwired: 2 out]
          }
        }
      }
      event "公式一键写入": Value Change {
        n292 = event-data() -> ()  [unwired: 1 in, 6 out]
        n293 = local read "公式"() -> (w530:cluster{"X^2":dbl, "X":dbl, "b":dbl})
        n294 = call "公式复合写入.vi"("公式"=w530) -> ()  [unwired: 11 in]
      }
      event "备用系数一键写入": Value Change {
        n295 = event-data() -> ()  [unwired: 1 in, 6 out]
        n296 = local read "备用系数"() -> (w531:T4)
        n297 = call "量程参数复合参数写入.vi"("备用系数"=w531) -> ()  [unwired: 11 in]
      }
      event "曲线模型": Value Change {
        n298 = event-data() -> ()  [unwired: 1 in, 6 out]
        n299 = Unbundle By Name("曲线模型") -> ("X^2"=w535:dbl, "X"=w534:dbl, "B"=w533:dbl)
        n300 = local read "公式"() -> (w537:cluster{"X^2":dbl, "X":dbl, "b":dbl})
        n301 = Bundle By Name(cluster=w537, "X^2"=w535, "X"=w534, "b"=w533) -> (w532:cluster{"X^2":dbl, "X":dbl, "b":dbl})
        n302 = local write "公式"(w532) -> ()
      }
      event "质控参数设置": Value Change {
        n303 = event-data() -> ()  [unwired: 1 in, 6 out]
        n304 = global read "总磷总氮断电保存全局变量.vi" "质控参数设置"() -> (w538:T24)
        n305 = call "总磷总氮质控参数设置.vi"("质控参数设置"=w538) -> ("输出簇"=w539:T25)  [unwired: 10 in]
        n306 = Unbundle By Name(w539) -> ("确定"=w540:bool)
        n307 = case shown="真" w540 {
          tunnel: w539 -> [_ w542]
          tunnel: w538 -> [_ w541]
          frame False {
          }
          frame True {
            n308 = flat-sequence {
              tunnel: w542 -> [w553]
              tunnel: w541 -> [w552]
              frame #0 {
                n309 = Unbundle By Name(w553) -> ("总磷跨度值"=w551:dbl, "总磷零点标准液浓度"=w550:dbl, "总磷跨度标准液浓度"=w549:dbl, "总磷标准液标准浓度"=w548:dbl, "总氮跨度值"=w547:dbl, "总氮零点标准液浓度"=w546:dbl, "总氮跨度标准液浓度"=w545:dbl, "总氮标准液标准浓度"=w544:dbl)
                n310 = Bundle By Name(cluster=w552, "总磷跨度值"=w551, "总磷零点标准液浓度"=w550, "总磷跨度标准液浓度"=w549, "总磷标准液标准浓度"=w548, "总氮跨度值"=w547, "总氮零点标准液浓度"=w546, "总氮跨度标准液浓度"=w545, "总氮标准液标准浓度"=w544) -> (w543:T24)
                n311 = global write "总磷总氮断电保存全局变量.vi" "质控参数设置"(w543) -> ()
              }
              frame #1 {
                n312 = call <vilib>:"Application Directory.vi"() -> ("Application Directory"=w567:path)
                n313 = Build Path(base path=w567, name or relative path="data\\sys.ini" ("名称或相对路径")) -> (appended path=w565:path)
                n314 = call <vilib>:"Open Config Data.vi"("configuration file path"=w565) -> ("error out"=w561:errorcluster, "refnum"=w564:T15)  [unwired: 8 in, 1 out]
                n315 = vi-ref "总磷总氮断电保存全局变量.vi"() -> (w563:refnum<vi>)
                n316 = call <userlib>:"Write Panel to INI__ogtk.vi"("error in (no error)"=w561, "VI ref"=w563, "refnum"=w564) -> ("error out"=w560:errorcluster, "refnum out"=w562:T15)  [unwired: 7 in]
                n317 = call <vilib>:"Close Config Data.vi"("error in (no error)"=w560, "refnum"=w562) -> ("error out"=w555:errorcluster, "file path"=w554:path)  [unwired: 8 in]
                n318 = Open/Create/Replace File(file path (use dialog)=w554, error in=w555) -> (refnum out=w558:refnum<file>, error out=w559:errorcluster)  [unwired: 4 in, 1 out]
                n319 = Flush File(refnum=w558, error in=w559) -> (refnum out=w557:refnum<file>, error out=w556:errorcluster)
                n320 = Close File(refnum=w557, error in=w556) -> ()  [unwired: 2 out]
              }
            }
          }
        }
      }
      event "总氮参数设置": Value Change {
        n321 = event-data() -> ()  [unwired: 1 in, 6 out]
        n322 = global read "总磷总氮断电保存全局变量.vi" "总氮仪器参数"() -> (w569:T26)
        n323 = call "仪器参数设置.vi"("氨氮仪器参数"=w569) -> ("仪器参数设置输出"=w568:T27)  [unwired: 10 in]
        n324 = Unbundle By Name(w568) -> ("确定"=w570:bool)
        n325 = case shown="真" w570 {
          tunnel: w568 -> [_ w572]
          tunnel: w569 -> [_ w571]
          frame False {
          }
          frame True {
            n326 = flat-sequence {
              tunnel: w572 -> [w588]
              tunnel: w571 -> [w587]
              frame #0 {
                n327 = Unbundle By Name(w588) -> ("测量量程"=w586:dbl, "测量精度"=w585:dbl, "测量间隔"=w584:dbl, "消解温度"=w583:dbl, "消解时长"=w582:dbl, "空白校准时间"=w581:timestamp, "曲线截距"=w580:dbl, "曲线斜率"=w579:dbl, "测量检出限"=w577:dbl, "测量信号值"=w576:dbl, "线性相关系数"=w575:dbl, "二次多项式系数"=w574:dbl, "标样校准时间"=w573:timestamp)
                n328 = Bundle By Name(cluster=w587, "测量量程"=w586, "测量精度"=w585, "测量间隔"=w584, "消解温度"=w583, "消解时长"=w582, "空白校准时间"=w581, "曲线截距"=w580, "曲线斜率"=w579, "测量检出限"=w577, "测量信号值"=w576, "线性相关系数"=w575, "二次多项式系数"=w574, "标样校准时间"=w573) -> (w578:T26)
                n329 = global write "总磷总氮断电保存全局变量.vi" "总氮仪器参数"(w578) -> ()
              }
              frame #1 {
                n330 = call <vilib>:"Application Directory.vi"() -> ("Application Directory"=w602:path)
                n331 = Build Path(base path=w602, name or relative path="data\\sys.ini" ("名称或相对路径")) -> (appended path=w600:path)
                n332 = call <vilib>:"Open Config Data.vi"("configuration file path"=w600) -> ("error out"=w596:errorcluster, "refnum"=w599:T15)  [unwired: 8 in, 1 out]
                n333 = vi-ref "总磷总氮断电保存全局变量.vi"() -> (w598:refnum<vi>)
                n334 = call <userlib>:"Write Panel to INI__ogtk.vi"("error in (no error)"=w596, "VI ref"=w598, "refnum"=w599) -> ("error out"=w595:errorcluster, "refnum out"=w597:T15)  [unwired: 7 in]
                n335 = call <vilib>:"Close Config Data.vi"("error in (no error)"=w595, "refnum"=w597) -> ("error out"=w590:errorcluster, "file path"=w589:path)  [unwired: 8 in]
                n336 = Open/Create/Replace File(file path (use dialog)=w589, error in=w590) -> (refnum out=w593:refnum<file>, error out=w594:errorcluster)  [unwired: 4 in, 1 out]
                n337 = Flush File(refnum=w593, error in=w594) -> (refnum out=w592:refnum<file>, error out=w591:errorcluster)
                n338 = Close File(refnum=w592, error in=w591) -> ()  [unwired: 2 out]
              }
            }
          }
        }
      }
      event "总磷参数设置": Value Change {
        n339 = event-data() -> ()  [unwired: 1 in, 6 out]
        n340 = global read "总磷总氮断电保存全局变量.vi" "总磷仪器参数"() -> (w604:T26)
        n341 = call "仪器参数设置.vi"("氨氮仪器参数"=w604) -> ("仪器参数设置输出"=w603:T27)  [unwired: 10 in]
        n342 = Unbundle By Name(w603) -> ("确定"=w605:bool)
        n343 = case shown="真" w605 {
          tunnel: w603 -> [_ w607]
          tunnel: w604 -> [_ w606]
          frame False {
          }
          frame True {
            n344 = flat-sequence {
              tunnel: w607 -> [w623]
              tunnel: w606 -> [w622]
              frame #0 {
                n345 = Unbundle By Name(w623) -> ("测量量程"=w621:dbl, "测量精度"=w620:dbl, "测量间隔"=w619:dbl, "消解温度"=w618:dbl, "消解时长"=w617:dbl, "空白校准时间"=w616:timestamp, "曲线截距"=w615:dbl, "曲线斜率"=w614:dbl, "测量检出限"=w612:dbl, "测量信号值"=w611:dbl, "线性相关系数"=w610:dbl, "二次多项式系数"=w609:dbl, "标样校准时间"=w608:timestamp)
                n346 = Bundle By Name(cluster=w622, "测量量程"=w621, "测量精度"=w620, "测量间隔"=w619, "消解温度"=w618, "消解时长"=w617, "空白校准时间"=w616, "曲线截距"=w615, "曲线斜率"=w614, "测量检出限"=w612, "测量信号值"=w611, "线性相关系数"=w610, "二次多项式系数"=w609, "标样校准时间"=w608) -> (w613:T26)
                n347 = global write "总磷总氮断电保存全局变量.vi" "总磷仪器参数"(w613) -> ()
              }
              frame #1 {
                n348 = call <vilib>:"Application Directory.vi"() -> ("Application Directory"=w637:path)
                n349 = Build Path(base path=w637, name or relative path="data\\sys.ini" ("名称或相对路径")) -> (appended path=w635:path)
                n350 = call <vilib>:"Open Config Data.vi"("configuration file path"=w635) -> ("error out"=w631:errorcluster, "refnum"=w634:T15)  [unwired: 8 in, 1 out]
                n351 = vi-ref "总磷总氮断电保存全局变量.vi"() -> (w633:refnum<vi>)
                n352 = call <userlib>:"Write Panel to INI__ogtk.vi"("error in (no error)"=w631, "VI ref"=w633, "refnum"=w634) -> ("error out"=w630:errorcluster, "refnum out"=w632:T15)  [unwired: 7 in]
                n353 = call <vilib>:"Close Config Data.vi"("error in (no error)"=w630, "refnum"=w632) -> ("error out"=w625:errorcluster, "file path"=w624:path)  [unwired: 8 in]
                n354 = Open/Create/Replace File(file path (use dialog)=w624, error in=w625) -> (refnum out=w628:refnum<file>, error out=w629:errorcluster)  [unwired: 4 in, 1 out]
                n355 = Flush File(refnum=w628, error in=w629) -> (refnum out=w627:refnum<file>, error out=w626:errorcluster)
                n356 = Close File(refnum=w627, error in=w626) -> ()  [unwired: 2 out]
              }
            }
          }
        }
      }
      event "总磷自动测试量程配置", "总氮自动测试量程配置": Value Change {
        n357 = event-data() -> ()  [unwired: 1 in, 6 out]
        n358 = flat-sequence {
          frame #0 {
            n359 = global write "总磷总氮断电保存全局变量.vi" "总氮自动测试量程配置"("总氮自动测试量程配置") -> ()
            n360 = global write "总磷总氮断电保存全局变量.vi" "总磷自动测试量程配置"("总磷自动测试量程配置") -> ()
          }
          frame #1 {
            n361 = call <vilib>:"Application Directory.vi"() -> ("Application Directory"=w653:path)
            n362 = Build Path(base path=w653, name or relative path="data\\sys.ini" ("名称或相对路径")) -> (appended path=w651:path)
            n363 = call <vilib>:"Open Config Data.vi"("configuration file path"=w651) -> ("error out"=w647:errorcluster, "refnum"=w650:T15)  [unwired: 8 in, 1 out]
            n364 = vi-ref "总磷总氮断电保存全局变量.vi"() -> (w649:refnum<vi>)
            n365 = call <userlib>:"Write Panel to INI__ogtk.vi"("error in (no error)"=w647, "VI ref"=w649, "refnum"=w650) -> ("error out"=w646:errorcluster, "refnum out"=w648:T15)  [unwired: 7 in]
            n366 = call <vilib>:"Close Config Data.vi"("error in (no error)"=w646, "refnum"=w648) -> ("error out"=w641:errorcluster, "file path"=w640:path)  [unwired: 8 in]
            n367 = Open/Create/Replace File(file path (use dialog)=w640, error in=w641) -> (refnum out=w644:refnum<file>, error out=w645:errorcluster)  [unwired: 4 in, 1 out]
            n368 = Flush File(refnum=w644, error in=w645) -> (refnum out=w643:refnum<file>, error out=w642:errorcluster)
            n369 = Close File(refnum=w643, error in=w642) -> ()  [unwired: 2 out]
          }
        }
      }
      event "手动启动": Value Change {
        n370 = event-data() -> ()  [unwired: 1 in, 6 out]
        n371 = call "总磷总氮启动参数对话框.vi"() -> ("确认"=w654:bool, "元素"=w655:cluster{"命令":string, "data":variant})  [unwired: 10 in]
        n372 = case shown="真" w654 {
          tunnel: w656 -> [_ w658]
          tunnel: w655 -> [_ w657]
          frame False {
          }
          frame True {
            n373 = Enqueue Element(queue=w658, element=w657) -> ()  [unwired: 2 in, 3 out]
          }
        }
      }
      event "单步测试": Value Change {
        w660 = u16 1 items=["总磷"=1, "氨氮"=3] ("站号")
        n374 = event-data() -> ()  [unwired: 1 in, 6 out]
        n375 = Bundle("站号"=w660, "总磷氨氮调试"="总磷氨氮调试") -> (w659:cluster{"站号":u16, "总磷氨氮调试":u16[]})  [unwired: 1 in]
        n376 = Bundle By Name(cluster=cluster{"命令":string, "data":variant} {"命令"="", "data"=variant} ("元素"), "命令"="debug", "data"=w659) -> (w662:cluster{"命令":string, "data":variant})
        n377 = Enqueue Element(queue=w665, element=w662) -> ()  [unwired: 2 in, 3 out]
      }
      event "停止": Value Change {
        n378 = event-data() -> ()  [unwired: 1 in, 6 out]
        n379 = Enqueue Element(queue=w669, element=cluster{"命令":string, "data":variant} {"命令"="启动", "data"=variant(cluster{"站号":u16, "控制命令输出":u16[]} {"站号"=1, "控制命令输出"=[2816]})} ("元素")) -> (queue out=w666:refnum<queue>)  [unwired: 2 in, 2 out]
        n380 = Enqueue Element(queue=w666, element=cluster{"命令":string, "data":variant} {"命令"="启动", "data"=variant(cluster{"站号":u16, "控制命令输出":u16[]} {"站号"=2, "控制命令输出"=[2816]})} ("元素")) -> ()  [unwired: 2 in, 3 out]
      }
      event "设置": Value Change {
        n381 = event-data() -> ()  [unwired: 1 in, 6 out]
        n382 = property on="窗格" class="Pane"("Origin"=T16 {"Horizontal"=0, "Vertical"=628} ("原点")) -> ()  [unwired: 2 in, 2 out]
      }
      event "返回": Value Change {
        n383 = event-data() -> ()  [unwired: 1 in, 6 out]
        n384 = property on="窗格" class="Pane"("Origin"=T16 {"Horizontal"=0, "Vertical"=0} ("原点")) -> ()  [unwired: 2 in, 2 out]
      }
      event "公式.X^2", "公式.X", "公式.b", "量程切换阈值.阈值", "量程切换阈值.标液浓度", "备用系数.量程上限", "备用系数.量程下限", "备用系数.检出限", "备用系数.精度": Mouse Down {
        n385 = event-data() -> ("CtlRef"=w675:refnum<vi>)  [unwired: 1 in, 5 out]
        n386 = property class="DigNum (严格)"(reference=w675) -> (reference out=w673:refnum<vi>, "Value"=w674:dbl)  [unwired: 1 in, 1 out]
        n387 = call "数字键盘.vi"("OldNumber"=w674) -> ("NewNumber"=w672:dbl)
        n388 = property class="DigNum (严格)"(reference=w673, "Val(Sgnl)"=w672) -> ()  [unwired: 1 in, 2 out]
      }
      event "读公式": Value Change {
        n389 = event-data() -> ()  [unwired: 1 in, 6 out]
        n390 = property class="Enum (严格)"(reference=w683) -> ("Value"=w682:enum16{"总磷", "总氮"})  [unwired: 1 in, 2 out]
        n391 = property class="Enum (严格)"(reference=w684) -> ("Value"=w681:enum16{"水样测量", "零点核查", "跨度核查", "标样核查", "加标回收"})  [unwired: 1 in, 2 out]
        n392 = property class="Enum (严格)"(reference=w685) -> ("Value"=w680:enum16{"低量程", "高量程"})  [unwired: 1 in, 2 out]
        n393 = call "总磷总氮公式读取.vi"("量程"=w680, "测量模式"=w681, "测量参数"=w682) -> ("error out"=w677:errorcluster, "公式"=w678:cluster{"X^2":dbl, "X":dbl, "b":dbl})  [unwired: 7 in]
        n394 = property class="Clust (严格)"(reference=w679, "Value"=w678) -> ()  [unwired: 1 in, 2 out]
        n395 = case shown="错误" w677 {
          tunnel: ["读取成功" ("消息") "读取失败" ("消息")] -> w676
          frame No Error {
          }
          frame Error {
          }
        }
        n396 = One Button Dialog(message=w676) -> ()  [unwired: 1 in, 1 out]
      }
      event "写公式": Value Change {
        n397 = event-data() -> ()  [unwired: 1 in, 6 out]
        n398 = call "总磷总氮公式写入.vi"("公式"="公式", "量程"="量程下拉列表", "测量模式"="测量模式下拉列表", "测量参数"="参数下拉列表") -> ("error out"=w692:errorcluster)  [unwired: 7 in]
        n399 = case shown="无错误" w692 {
          tunnel: ["写入成功" ("消息") "写入失败" ("消息")] -> w693
          tunnel: "公式" -> [w702 _]
          tunnel: "测量模式下拉列表" -> [w700 _]
          tunnel: "量程下拉列表" -> [w698 _]
          tunnel: "参数下拉列表" -> [w697 _]
          frame No Error {
            n400 = Equal?(x=w700, y=enum16{"水样测量", "零点核查", "跨度核查", "标样核查", "加标回收"}."水样测量" ("测量模式下拉列表")) -> (x = y?=w696:bool)
            n401 = Equal?(x=w698, y=enum16{"低量程", "高量程"}."低量程" ("量程下拉列表")) -> (x = y?=w695:bool)
            n402 = And(x=w696, y=w695) -> (x .and. y?=w694:bool)
            n403 = case shown="真" w694 {
              tunnel: w702 -> [_ w705]
              tunnel: w697 -> [_ w704]
              frame False {
              }
              frame True {
                n404 = case shown="\"总磷\", 默认" w704 {
                  tunnel: w705 -> [w706 w712]
                  frame "总磷", Default {
                    n405 = Unbundle By Name(w706) -> ("X^2"=w709:dbl, "X"=w708:dbl, "b"=w707:dbl)
                    n406 = global read "总磷总氮断电保存全局变量.vi" "总磷仪器参数"() -> (w710:T26)
                    n407 = Bundle By Name(cluster=w710, "曲线截距"=w707, "曲线斜率"=w708, "二次多项式系数"=w709) -> (w711:T26)
                    n408 = global write "总磷总氮断电保存全局变量.vi" "总磷仪器参数"(w711) -> ()
                  }
                  frame "总氮" {
                    n409 = Unbundle By Name(w712) -> ("X^2"=w715:dbl, "X"=w714:dbl, "b"=w713:dbl)
                    n410 = global read "总磷总氮断电保存全局变量.vi" "总氮仪器参数"() -> (w716:T26)
                    n411 = Bundle By Name(cluster=w716, "曲线截距"=w713, "曲线斜率"=w714, "二次多项式系数"=w715) -> (w717:T26)
                    n412 = global write "总磷总氮断电保存全局变量.vi" "总氮仪器参数"(w717) -> ()
                  }
                }
              }
            }
          }
          frame Error {
          }
        }
        n413 = One Button Dialog(message=w693) -> ()  [unwired: 1 in, 1 out]
      }
      event "量程切换阈值读取": Value Change {
        n414 = event-data() -> ()  [unwired: 1 in, 6 out]
        n415 = property class="Enum (严格)"(reference=w726) -> ("Value"=w725:enum16{"总磷", "总氮"})  [unwired: 1 in, 2 out]
        n416 = property class="Enum (严格)"(reference=w727) -> ("Value"=w724:enum16{"水样测量", "零点核查", "跨度核查", "标样核查", "加标回收"})  [unwired: 1 in, 2 out]
        n417 = property class="Enum (严格)"(reference=w728) -> ("Value"=w723:enum16{"低量程", "高量程"})  [unwired: 1 in, 2 out]
        n418 = call "总磷总氮量程读取.vi"("量程"=w723, "测量模式"=w724, "测量参数"=w725) -> ("error out"=w719:errorcluster, "量程切换阈值"=w721:cluster{"阈值":dbl, "标液浓度":dbl})  [unwired: 7 in]
        n419 = property class="Clust (严格)"(reference=w722, "Value"=w721) -> ()  [unwired: 1 in, 2 out]
        n420 = case shown="错误" w719 {
          tunnel: ["读取成功" ("消息") "读取失败" ("消息")] -> w720
          frame No Error {
          }
          frame Error {
          }
        }
        n421 = One Button Dialog(message=w720) -> ()  [unwired: 1 in, 1 out]
      }
      event "量程切换阈值写入": Value Change {
        n422 = event-data() -> ()  [unwired: 1 in, 6 out]
        n423 = property class="Enum (严格)"(reference=w739) -> ("Value"=w736:enum16{"总磷", "总氮"})  [unwired: 1 in, 2 out]
        n424 = property class="Enum (严格)"(reference=w738) -> ("Value"=w735:enum16{"水样测量", "零点核查", "跨度核查", "标样核查", "加标回收"})  [unwired: 1 in, 2 out]
        n425 = property class="Enum (严格)"(reference=w737) -> ("Value"=w734:enum16{"低量程", "高量程"})  [unwired: 1 in, 2 out]
        n426 = call "总磷总氮量程写入.vi"("量程切换阈值"="量程切换阈值", "量程"=w734, "测量模式"=w735, "测量参数"=w736) -> ("error out"=w731:errorcluster)  [unwired: 7 in]
        n427 = case shown="无错误" w731 {
          tunnel: ["写入成功" ("消息") "写入失败" ("消息")] -> w732
          frame No Error {
          }
          frame Error {
          }
        }
        n428 = One Button Dialog(message=w732) -> ()  [unwired: 1 in, 1 out]
      }
      event "备用系数读取": Value Change {
        n429 = event-data() -> ()  [unwired: 1 in, 6 out]
        n430 = property class="Enum (严格)"(reference=w751) -> ("Value"=w750:enum16{"总磷", "总氮"})  [unwired: 1 in, 2 out]
        n431 = property class="Enum (严格)"(reference=w744) -> ("Value"=w743:enum16{"水样测量", "零点核查", "跨度核查", "标样核查", "加标回收"})  [unwired: 1 in, 2 out]
        n432 = property class="Enum (严格)"(reference=w745) -> ("Value"=w742:enum16{"低量程", "高量程"})  [unwired: 1 in, 2 out]
        n433 = call "总磷总氮备用系数读取.vi"("量程"=w742, "测量模式"=w743, "测量参数"=w750) -> ("error out"=w746:errorcluster, "备用系数"=w748:T4)  [unwired: 7 in]
        n434 = property class="Clust (严格)"(reference=w749, "Value"=w748) -> ()  [unwired: 1 in, 2 out]
        n435 = case shown="错误" w746 {
          tunnel: ["读取成功" ("消息") "读取失败" ("消息")] -> w747
          frame No Error {
          }
          frame Error {
          }
        }
        n436 = One Button Dialog(message=w747) -> ()  [unwired: 1 in, 1 out]
      }
      event "备用系数写入": Value Change {
        n437 = event-data() -> ()  [unwired: 1 in, 6 out]
        n438 = property class="Enum (严格)"(reference=w762) -> ("Value"=w761:enum16{"总磷", "总氮"})  [unwired: 1 in, 2 out]
        n439 = property class="Enum (严格)"(reference=w757) -> ("Value"=w755:enum16{"水样测量", "零点核查", "跨度核查", "标样核查", "加标回收"})  [unwired: 1 in, 2 out]
        n440 = property class="Enum (严格)"(reference=w756) -> ("Value"=w754:enum16{"低量程", "高量程"})  [unwired: 1 in, 2 out]
        n441 = call "总磷总氮备用系数写入.vi"("备用系数"="备用系数", "量程"=w754, "测量模式"=w755, "测量参数"=w761) -> ("error out"=w758:errorcluster)  [unwired: 7 in]
        n442 = case shown="无错误" w758 {
          tunnel: ["写入成功" ("消息") "写入失败" ("消息")] -> w759
          frame No Error {
          }
          frame Error {
          }
        }
        n443 = One Button Dialog(message=w759) -> ()  [unwired: 1 in, 1 out]
      }
    }
  }
